vi "[Backup]BeamScanner.vi"() -> ()   [LabVIEW 2016]
uses:
  C:/Program Files/Ocean Optics/OmniDriver/OOI_HOME/NETOmniDriver-NET40.dll
  Program Files/Ocean Optics/OmniDriver/OOI_HOME/NETOmniDriver-NET40.dll
  <vilib>/DAQmx/write.llb/DAQmx Write (Digital Bool 1Line 1Point).vi
  <vilib>/DAQmx/write.llb/DAQmx Write (Analog DBL 1Chan 1Samp).vi
  <vilib>/DAQmx/write.llb/DAQmx Write (Analog 1D DBL NChan 1Samp).vi
  <vilib>/DAQmx/write.llb/DAQmx Write (Analog 2D DBL NChan NSamp).vi
  <vilib>/Analysis/baseanly.llb/Mean (DBL).vi
  <vilib>/DAQmx/read.llb/DAQmx Read (Raw 1D I16).vi
  <vilib>/DAQmx/create/channels.llb/DAQmx Create Channel (DO-Digital Output).vi
  <vilib>/DAQmx/miscellaneous.llb/DAQmx Fill In Error Info.vi
  <vilib>/DAQmx/create/channels.llb/DAQmx Create Channel (AO-Voltage-Basic).vi
  resources/MotorPosition.vi
  <vilib>/DAQmx/create/channels.llb/DAQmx Create Channel (AI-Voltage-Basic).vi
  <vilib>/DAQmx/configure/timing.llb/DAQmx Timing (Sample Clock).vi
  <vilib>/DAQmx/configure/trigger.llb/DAQmx Start Trigger (Digital Edge).vi
  <vilib>/Analysis/NI_AALBase.lvlib
  <resource>/objmgr/daqmx.rc
panel:
  in  "OCM Setup":bool
  in  "Home X":dbl=-121.7
  in  "Home  Y":dbl=-91.8
  in  "sampling rate (ADC)":u32(ring)=1250000 items=["500000"=500000, "750000"=750000, "1000000"=1000000, "1250000"=1250000]
  in  "Intgration time [us]":u32=44444 min=7000 max=10000000 step=1
  in  "Wavelength max":dbl=761.0 min=200.0 max=1100.0 step=1.0
  in  "Wavelength min":dbl=374.0 min=200.0 max=1100.0 step=1.0 format="%#.4g"
  out "spectral image":u32[][][](array[numeric])
  out "read task":refnum<k21>
  out "write task":refnum<k21>
  in  "Detector":u16(ring) items=["PMT", "QEPro", "Basler OCM"]
  out "scanning waveforms":dbl[][](array[numeric])
  out "Retrace":dbl[][](array[numeric])
  in  "Move to z":bool
  out "z-Position":sgl format="%.2g"
  out "xy-Position [µm]":sgl[](array[numeric]) min=0 max=500
  in  "Thrown samples":i16=500
  in  "Throw away":bool
  out "Samples/Pixel":u32
  in  "PMT output range":dbl(ring)=10.0 items=["-0,1V – 0,1V"=0.1, "-0,2V – 0,2V"=0.2, "-0,5V – 0,5V"=0.5, "-1V – 1V"=1.0, "-2V – 2V"=2.0, "-5V – 5V"=5.0, "-10V – 10V"=10.0]
  out "Time of last scan memory":string
  out "Info File contents memory":string
  out "Info File contents":string
  out "Time per line [s]":dbl format="%#.1g"
  out "Time of last scan":string
  out "scaling factor (length/voltage)":dbl
  in  "Additional info":string
  in  "Save":bool
  in  "Quit":bool
  in  "PMT sensitivity":dbl min=-1989.12 max=1989.12 format="%#.2f"
  in  "requested z-Position":dbl min=0.0 max=10.0
  in  "# steps":u16=20 step=1 format="%#.0f"
  out "Duration (m.s)":string
  in  "Scanrate (pixels/s)":u32(ring)=10000 items=["250 kHz"=250000, "125 kHz"=125000, "50 kHz (!)"=50000, "25 kHz (!)"=25000, "10 kHz (?)"=10000, "5 kHz (?)"=5000, "2 kHz"=2000, "1 kHz"=1000, "500 Hz"=500, "200 Hz"=200, "100 Hz"=100]
  out "Optimal":string
  out "Optimal pixel size [nm]":dbl format="%#.0f"
  in  "NA":dbl=1.0 min=0.0
  in  "Swap Memory":bool
  out "Memory":dbl[][](graph)
  out "System":bool
  in  "Use white point":bool
  in  "Magnification":dbl=20.0
  in  "Go home":bool
  in  "Go to white point":bool
  in  "z-Maximum val":dbl min=0.0 max=500.0 format="%#.2f"
  in  "z-Minimum val":dbl min=0.0 max=500.0 format="%#.2f"
  in  "z-Stacking":bool
  in  "Step size":dbl=1.0 min=0.0
  in  "z-Minimum":dbl(slide) min=0.0 max=500.0 step=1.0 scale=0.0..500.0
  in  "z-Maximum":dbl(slide)=0.30612244897959184 min=96.0 max=500.0 step=1.0 scale=0.0..500.0
  out "Path":path
  in  "File identifier":string="unnamed_file"
  in  "Save Image":bool
  in  "Scan":bool
  in  "y-Offset":dbl min=-480.0 max=480.0 format="%#.2f"
  in  "x-Offset":dbl min=-480.0 max=480.0 format="%#.2f"
  in  "Field of View":dbl(ring)=0.471281296023564 items=["4x4 µm"=0.02945508100147275, "8x8 µm"=0.0589101620029455, "16x16 µm"=0.117820324005891, "32x32 µm"=0.235640648011782, "64x64 µm"=0.471281296023564, "128x128 µm"=0.942562592047128, "256x256 µm"=1.885125184094256, "512x512 µm"=3.770250368188512, "1024x1024 µm"=7.540500736377024, "0x0"=0.0]
  out "Image":dbl[][](graph)
  in  "Number of pixels":i32(ring)=128 items=["8x8"=8, "16x16"=16, "32x32"=32, "64x64"=64, "128x128"=128, "256x256"=256, "512x512"=512, "1024x1024"=1024, "optimal"=640]
  # "make setup button"
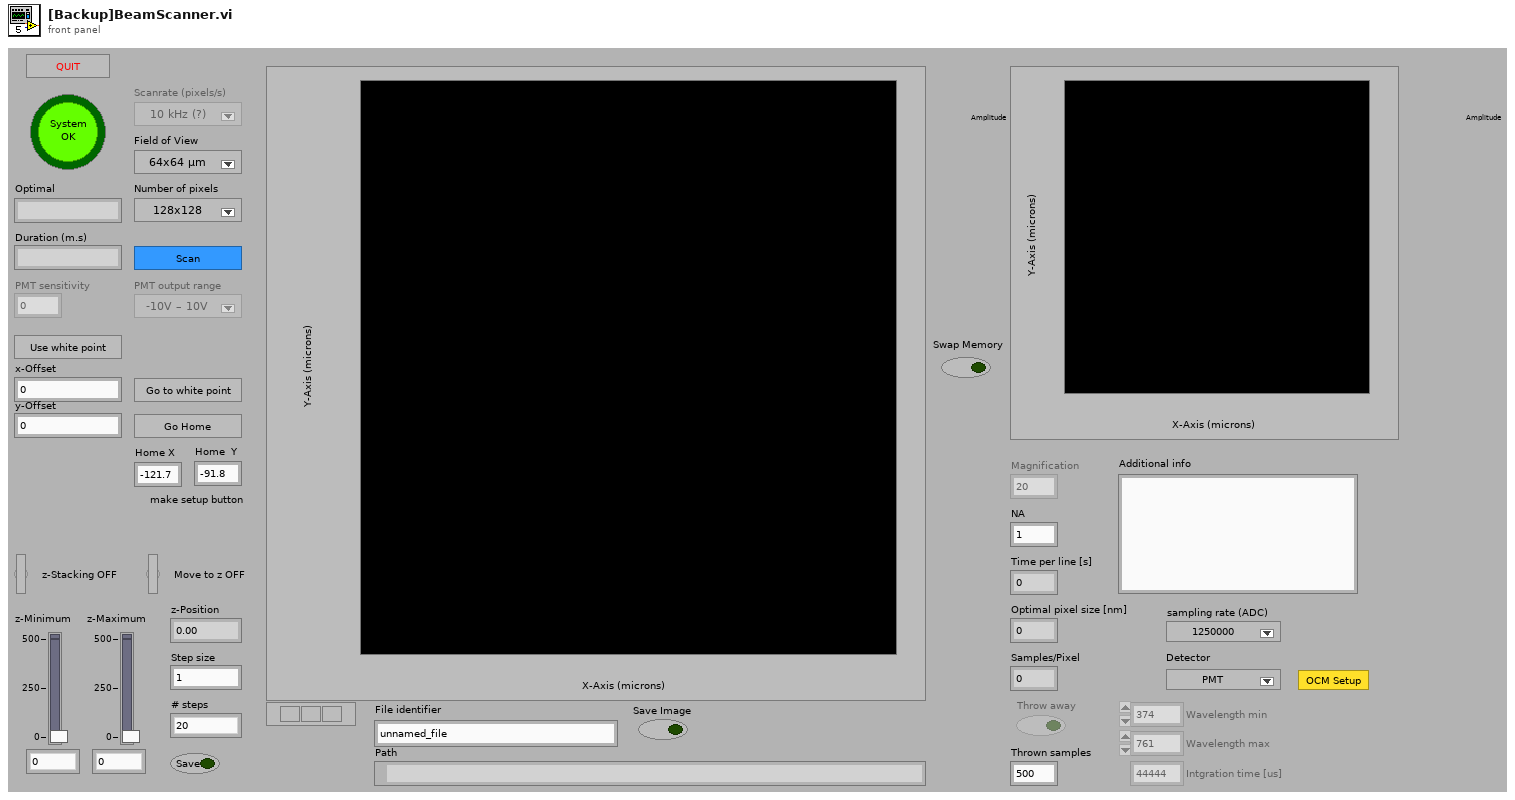
[diagram p1: front panel]
types:
  T1 = enum8{"Enabled", "Disabled", "Disabled and Grayed Out"}
  T2 = typedef "LVStringsAndValuesArrayTypeDef_DBL.ctl" = cluster{"String":string, "Value":dbl}[]
  T3 = typedef "LVStringsAndValuesArrayTypeDef_I32.ctl" = cluster{"String":string, "Value":i32}[]
  T4 = typedef "LVOffsetAndMultiplierTypeDef.ctl" = cluster{"Offset":dbl, "Multiplier":dbl}
  T5 = typedef "Maya2000 basic info.ctl" = cluster{"This instruments index":i32, "Name+SerialNumber":string, "Number Dark pixels":i32, "NumberOfPixels\nper spectrum":i32, "NumberOf Maya2000 instrm.":i32, "MaximumIntegrationTime\n[us]":i32, "MinimumIntegrationTime\n[us]":i32}
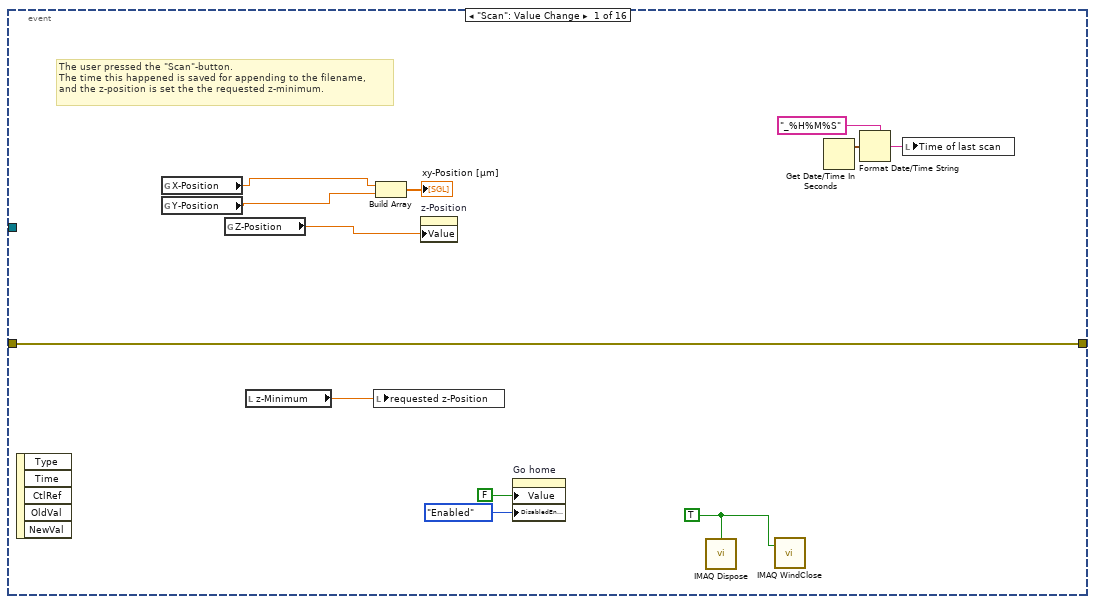
[diagram p2: hidden frame]
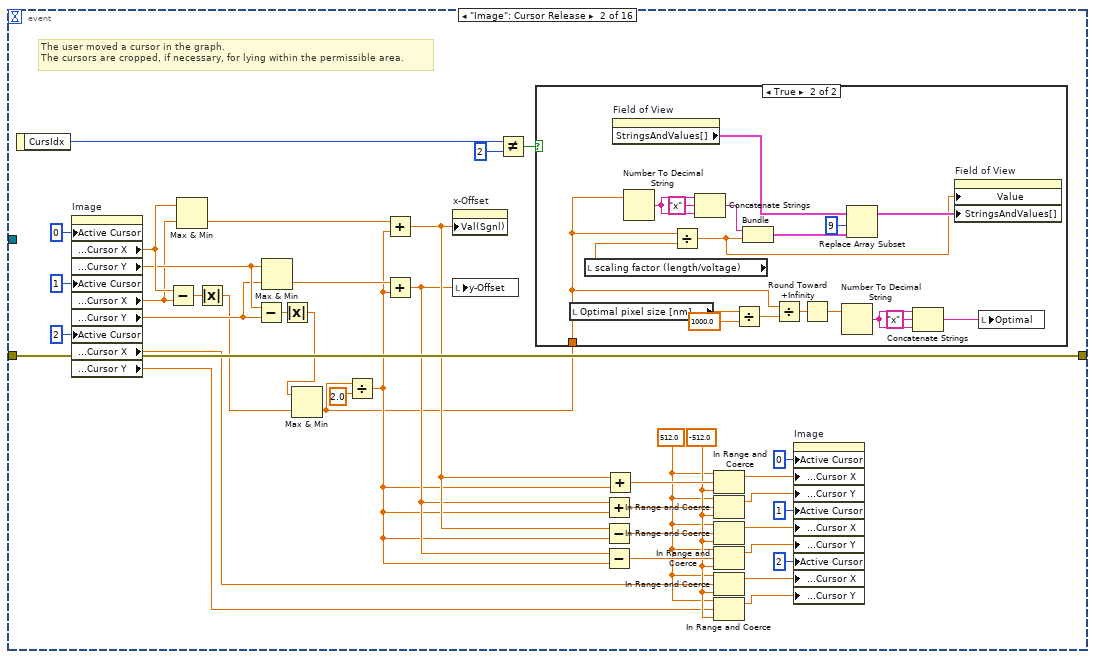
[diagram p3: hidden frame]
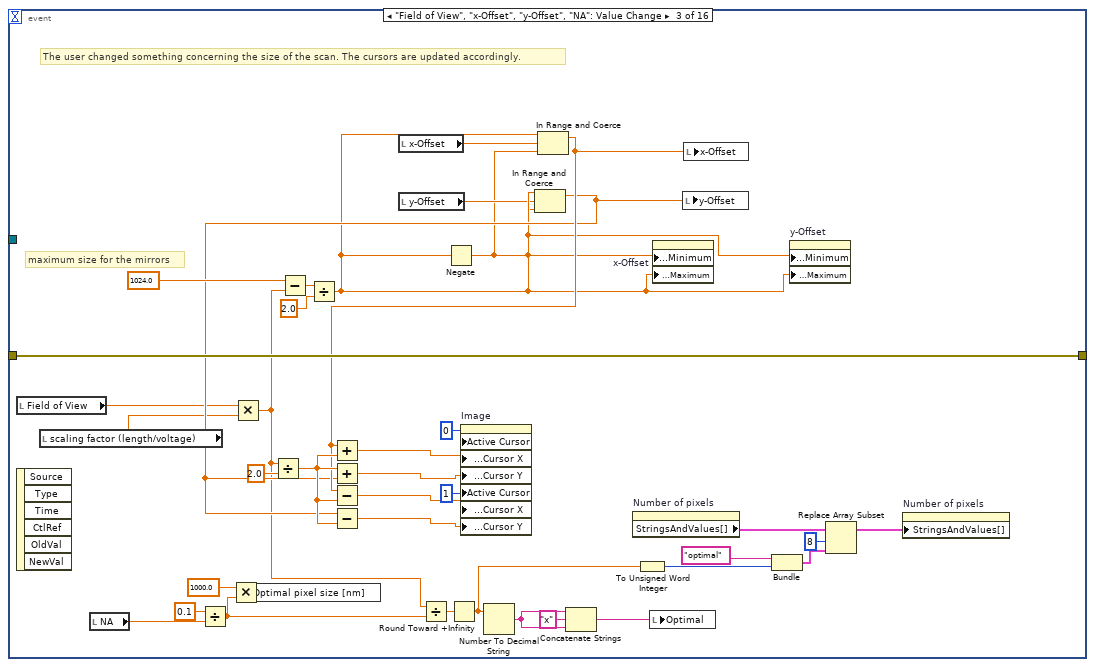
[diagram p5: hidden frame]
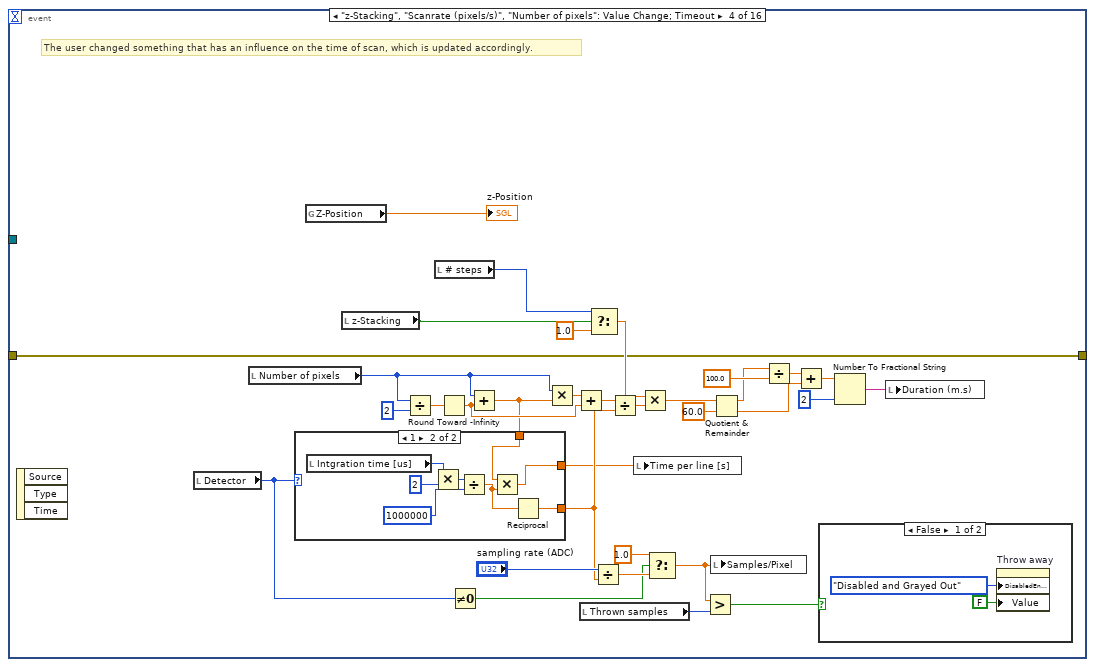
[diagram p6: hidden frame]
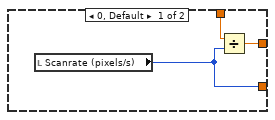
[diagram p7: hidden frame]
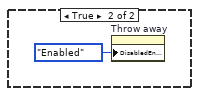
[diagram p8: hidden frame]
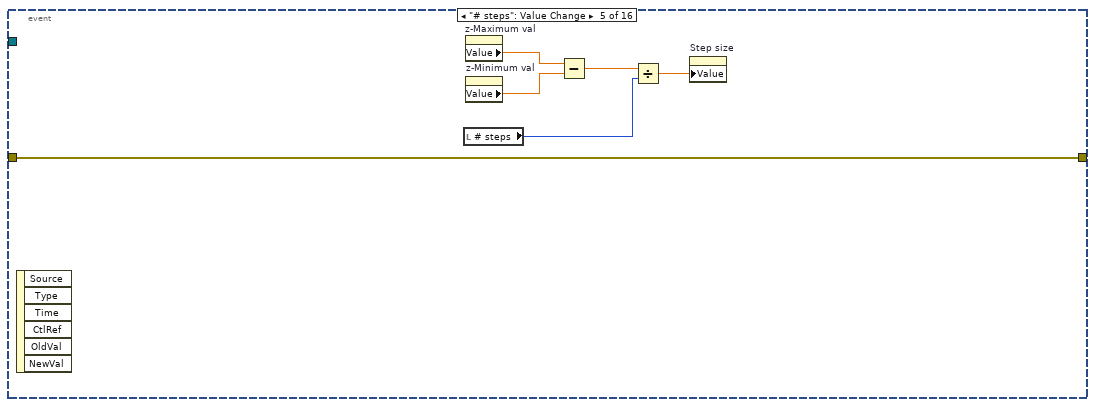
[diagram p9: hidden frame]
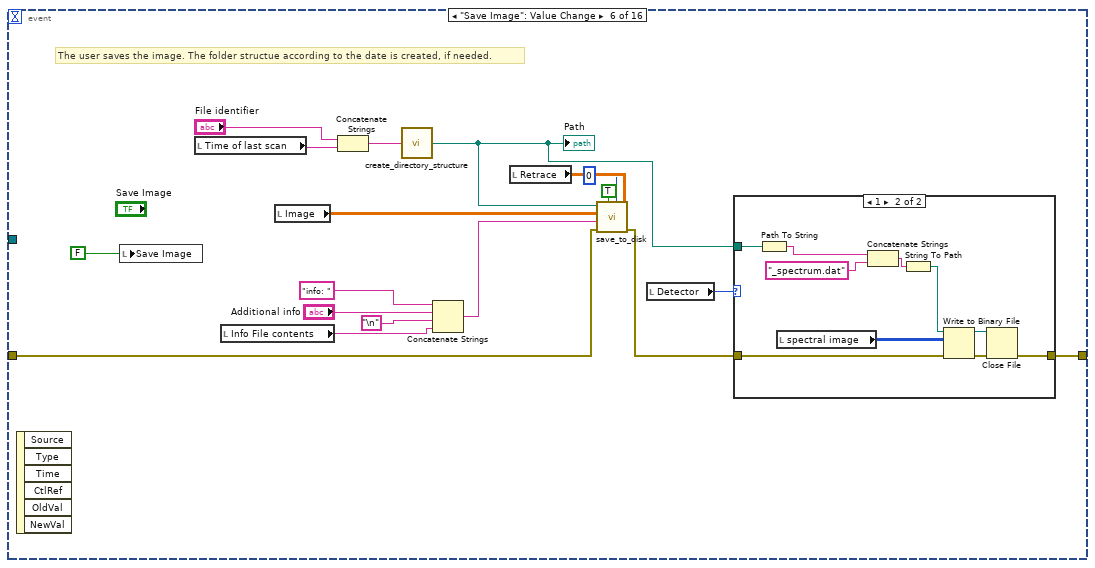
[diagram p10: hidden frame]
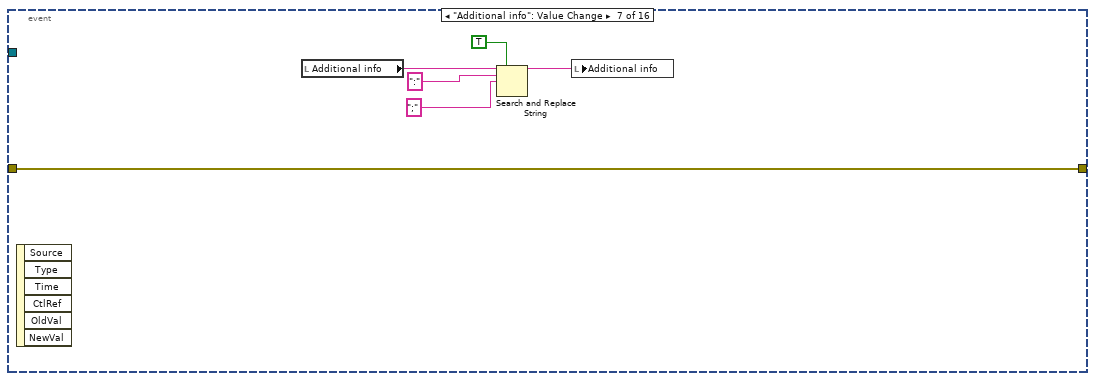
[diagram p12: hidden frame]
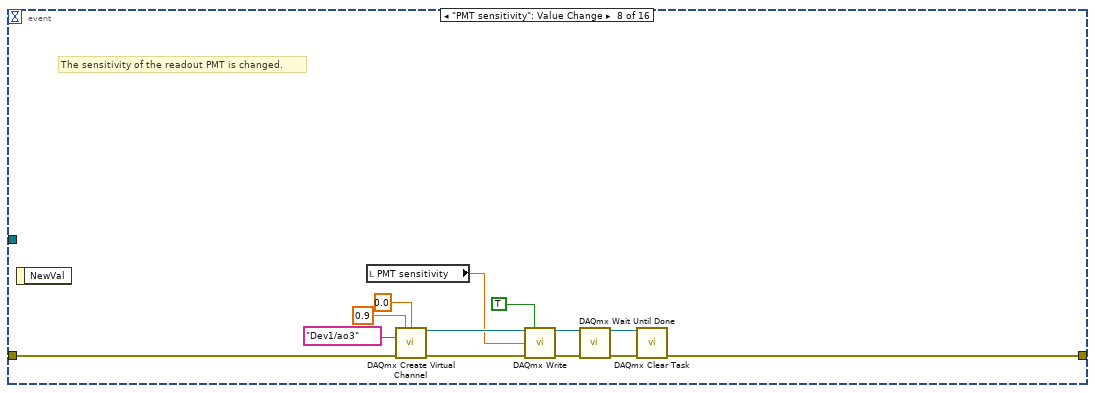
[diagram p13: hidden frame]
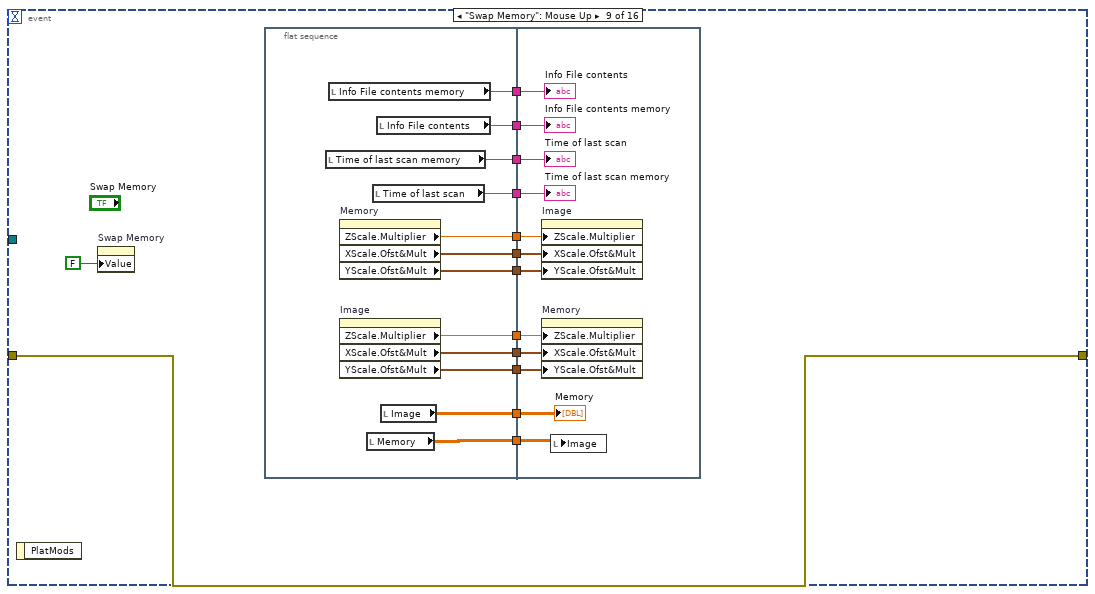
[diagram p14: hidden frame]
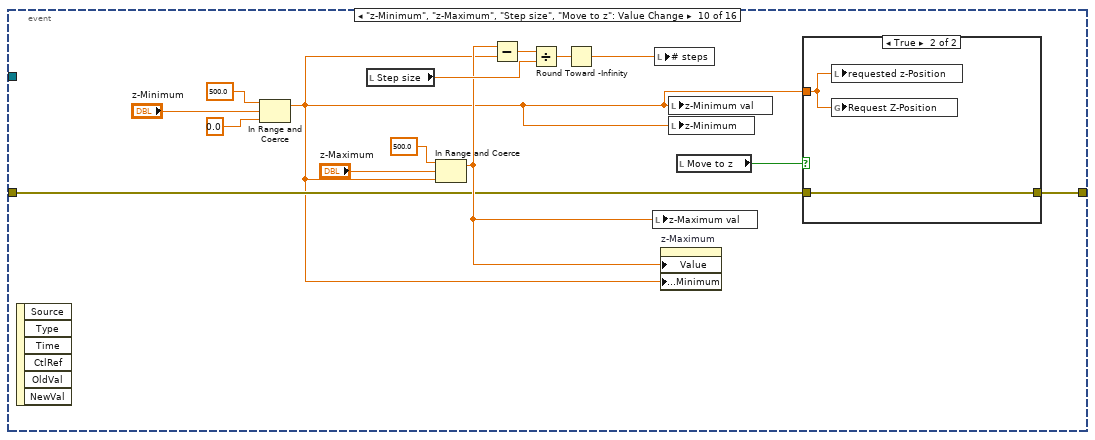
[diagram p15: hidden frame]
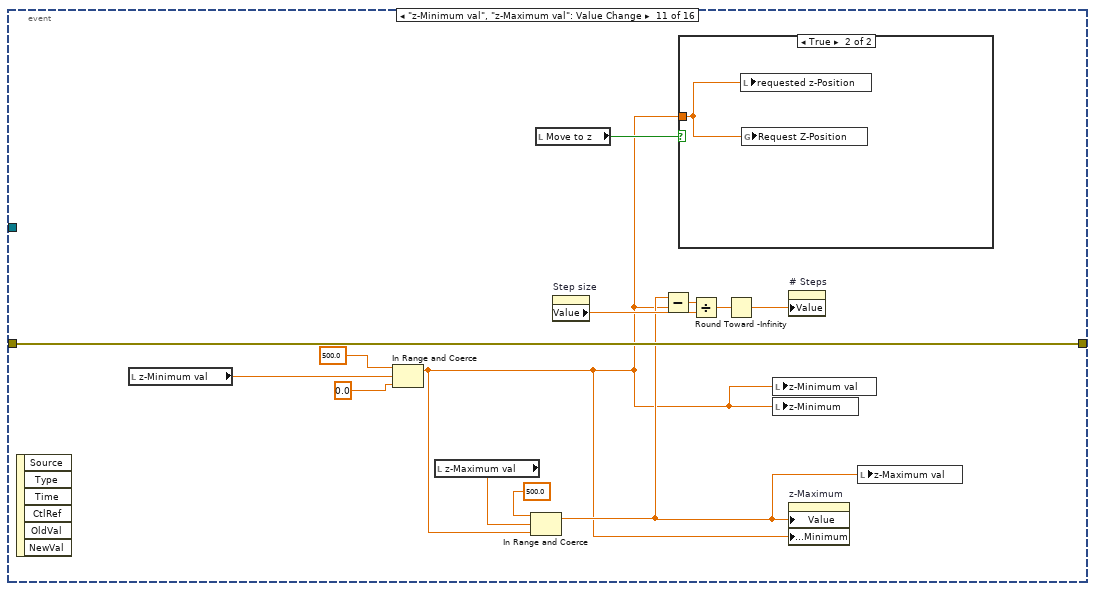
[diagram p17: hidden frame]
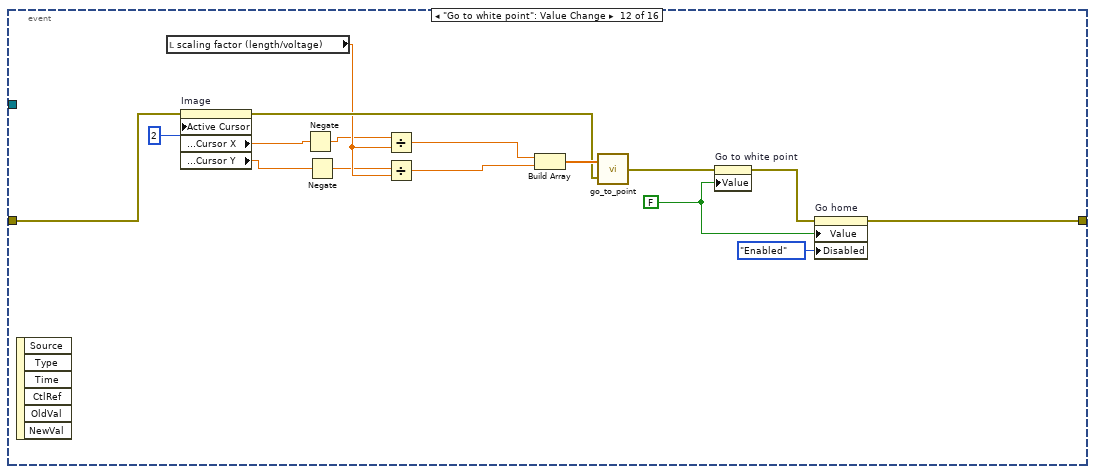
[diagram p19: hidden frame]
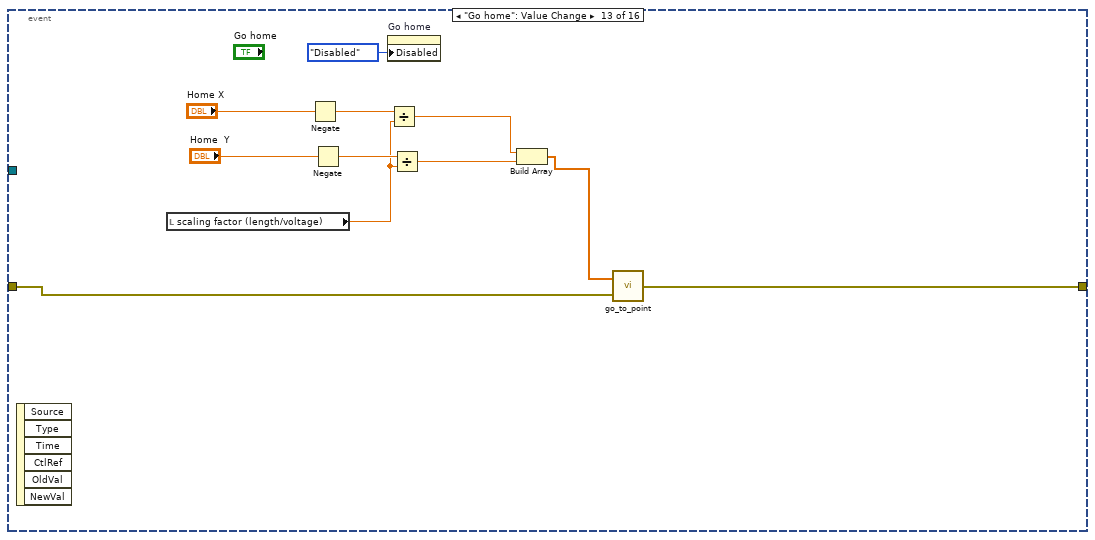
[diagram p20: hidden frame]
diagram:
  w2 = FALSE ("Visible")
  w24 = 0.0 ("y-Offset")
  w13 = FALSE ("System")
  # "These are local variable containers,\ninvisible to the user"
  # "Close the shutter"
  # "First, we initialise a few values, e.g.\nthe \"Save Image\" button is hidden,\nand the \"Scan\" button is set to false."
  n1 = call-poly <vilib>:"DAQmx Create Virtual Channel.vi"("lines"=tag "Dev1/port2/line0") -> ("task out"=w62:refnum<k21>, "error out"=w61:errorcluster)  [unwired: 13 in]
  n2 = property on="System" class="Bool (strict)"("Value"=TRUE ("System")) -> ()  [unwired: 2 in, 2 out]
  n3 = property on="Go to white point" class="Bool (strict)"("Value"=w13) -> ()  [unwired: 2 in, 2 out]
  n4 = property on="Quit" class="Bool (strict)"("Value"=w13) -> ()  [unwired: 2 in, 2 out]
  n5 = property on="Scan" class="Bool (strict)"("Value"=w13) -> ()  [unwired: 2 in, 2 out]
  n6 = property on="Go home" class="Bool (strict)"("Value"=w13, "DisabledEnum"=T1."Enabled" ("Disabled")) -> ()  [unwired: 2 in, 2 out]
  n7 = local write "x-Offset"(w24) -> ()
  n8 = local write "y-Offset"(w24) -> ()
  n9 = property on="OCM Setup" class="Bool"("Visible"=FALSE) -> ()  [unwired: 2 in, 2 out]
  n10 = call-poly <vilib>:"DAQmx Write.vi"("task/channels in"=w62, "data"=FALSE, "error in"=w61) -> ("task out"=w59:refnum<k21>, "error out"=w58:errorcluster)  [unwired: 10 in, 1 out]
  n11 = property on="Magnification" class="DigNum (strict)"("DisabledEnum"=T1."Disabled and Grayed Out" ("Disabled")) -> ()  [unwired: 2 in, 2 out]
  n12 = call <vilib>:"DAQmx Clear Task.vi"("task in"=w59, "error in"=w58) -> ("error out"=w46:errorcluster)  [unwired: 13 in]
  n13 = property on="write task" class="DAQmxName (strict)"("Visible"=w2) -> ()  [unwired: 2 in, 2 out]
  n14 = property on="read task" class="DAQmxName (strict)"("Visible"=w2) -> ()  [unwired: 2 in, 2 out]
  n15 = property on="scanning waveforms" class="Arr (strict)"("Visible"=w2) -> ()  [unwired: 2 in, 2 out]
  n16 = property on="Retrace" class="Arr (strict)"("Visible"=w2) -> ()  [unwired: 2 in, 2 out]
  n17 = property on="info file contents" class="Str"("Visible"=w2) -> ()  [unwired: 2 in, 2 out]
  n18 = property on="time of last scan" class="Str"("Visible"=w2) -> ()  [unwired: 2 in, 2 out]
  n19 = property on="info file contents memory" class="Str"("Visible"=w2) -> ()  [unwired: 2 in, 2 out]
  n20 = property on="time of last scan memory" class="Str"("Visible"=w2) -> ()  [unwired: 2 in, 2 out]
  n21 = property on="scaling factor (length/voltage)" class="DigNum (strict)"("Visible"=w2) -> ()  [unwired: 2 in, 2 out]
  n22 = property on="xy-Position [µm]" class="Arr (strict)"("Visible"=w2) -> ()  [unwired: 2 in, 2 out]
  n23 = property on="spectral image" class="Arr (strict)"("Visible"=w2) -> ()  [unwired: 2 in, 2 out]
  n24 = property on="requested z-Position" class="DigNum (strict)"("Visible"=w2) -> ()  [unwired: 2 in, 2 out]
  n25 = Divide(x=0.1, y="NA") -> (x/y=w35:dbl)
  n26 = call-poly <vilib>:"DAQmx Create Virtual Channel.vi"("maximum value"=0.9, "minimum value"=0.0, "physical channels"=tag "Dev1/ao3", "error in"=w46) -> ("task out"=w50:refnum<k21>, "error out"=w49:errorcluster)  [unwired: 10 in]
  n27 = Divide(x=2716.0, y="Magnification") -> (x/y=w20:dbl)
  "scaling factor (length/voltage)" <- w20
  n28 = Multiply(x=1000.0, y=w35) -> (x*y=→"Optimal pixel size [nm]":dbl)
  n29 = call-poly <vilib>:"DAQmx Write.vi"("task/channels in"=w50, "auto start"=TRUE, "data"="PMT sensitivity", "error in"=w49) -> ("task out"=w53:refnum<k21>, "error out"=w52:errorcluster)  [unwired: 9 in, 1 out]
  n30 = for {
    N: 8 -> [_]
    tunnel: [w77] -> w29 mode=indexing
    i -> [w84]
    n31 = Add(x=3, y=w84) -> (x+y=w81:i32)
    n32 = Scale By Power Of 2(n=w81, x=u16 1) -> (x*2^n=w78:u16)
    n33 = Format Into String(format string="%dx%d", w78, w78) -> (resulting string=w79:string)  [unwired: 2 in, 1 out]
    n34 = Bundle(w79, w78) -> (w77:cluster{string, u16})  [unwired: 1 in]
  }
  n35 = call <vilib>:"DAQmx Wait Until Done.vi"("task/channels in"=w53, "error in"=w52) -> ("task out"=w48:refnum<k21>, "error out"=w47:errorcluster)  [unwired: 12 in]
  n36 = Multiply(x=w20, y="Field of View") -> (x*y=w39:dbl)
  n37 = call <vilib>:"DAQmx Clear Task.vi"("task in"=w48, "error in"=w47) -> ("error out"=w45:errorcluster)  [unwired: 13 in]
  n38 = Divide(x=w39, y=w35) -> (x/y=w38:dbl)
  n39 = Build Array(tag "Dev1/ao0" ("physical channels"), tag "Dev1/ao1" ("physical channels")) -> (w74:tag[])
  n40 = Round Toward +Infinity(x=w38) -> (ceil(x): smallest int >= x=w31:dbl)
  n41 = call <vilib>:"DAQmx Flatten Channel String.vi"("names in"=w74, "error in"=w45) -> ("names out"=w73:string, "error out"=w72:errorcluster)  [unwired: 12 in]
  n42 = Number To Decimal String(number=w31) -> (decimal integer string=w36:string)  [unwired: 1 in]
  n43 = To Unsigned Word Integer(number=w31) -> (unsigned 16bit integer=w30:u16)
  n44 = call-poly <vilib>:"DAQmx Create Virtual Channel.vi"("physical channels"=w73, "error in"=w72) -> ("task out"=w70:refnum<k21>, "error out"=w69:errorcluster)  [unwired: 12 in]
  n45 = for {
    N: 9 -> [_]
    tunnel: w20 -> [w87]
    tunnel: [w86] -> w18 mode=indexing
    i -> [w91]
    n46 = Add(x=2, y=w91) -> (x+y=w93:i32)
    n47 = Scale By Power Of 2(n=w93, x=u16 1) -> (x*2^n=w88:u16)
    n48 = Divide(x=w88, y=w87) -> (x/y=w85:dbl)
    n49 = Format Into String(format string="%dx%d \\B5m", w88, w88) -> (resulting string=w89:string)  [unwired: 2 in, 1 out]
    n50 = Bundle(w89, w85) -> (w86:cluster{string, dbl})  [unwired: 1 in]
  }
  n51 = Concatenate Strings(w36, "x" ("string"), w36) -> (→"Optimal":string)
  n52 = call-poly <vilib>:"DAQmx Write.vi"("task/channels in"=w70, "data"=dbl[] [0.0, 0.0], "error in"=w69) -> ("task out"=w67:refnum<k21>, "error out"=w65:errorcluster)  [unwired: 10 in, 1 out]
  n53 = Bundle("string"="optimal", w30) -> (w28:cluster{"string":string, u16})  [unwired: 1 in]
  n54 = call <vilib>:"DAQmx Wait Until Done.vi"("task/channels in"=w67, "error in"=w65) -> ("task out"=w66:refnum<k21>, "error out"=w64:errorcluster)  [unwired: 12 in]
  n55 = Build Array (concatenate)(w29, w28) -> (w27:cluster{"string":string, u16}[])
  n56 = call <vilib>:"DAQmx Clear Task.vi"("task in"=w66, "error in"=w64) -> ("error out"=w5:errorcluster)  [unwired: 13 in]
  n57 = property on="Number of pixels" class="Ring (strict)"("StringsAndValues[]"=w27) -> ()  [unwired: 2 in, 2 out]
  n58 = Open VI Reference(vi path=path "kinesis/kinesis.vi", error in (no error)=w5) -> (vi reference=w11:refnum<vi>, error out=w10:errorcluster)  [unwired: 4 in]
  n59 = invoke class="VI" method="Run VI"(reference=w11, error in=w10, "Wait until done"=FALSE ("Wait Until Done")) -> (reference out=w8:refnum<vi>, error out=w7:errorcluster)  [unwired: 2 in, 3 out]
  n60 = Bundle("format string"="0x0", 0.0) -> (w17:cluster{"format string":string, dbl})  [unwired: 1 in]
  n61 = Build Array (concatenate)(w18, w17) -> (w14:cluster{"format string":string, dbl}[])
  n62 = property on="Field of View" class="Ring (strict)"("Strings And Values []"=w14) -> ()  [unwired: 2 in, 2 out]
  n63 = invoke class="VI" method="FP.Open"(reference=w8, error in=w7, "Activate"=TRUE ("Activate?")) -> (reference out=w3:refnum<vi>, error out=w4:errorcluster)  [unwired: 2 in, 3 out]
  n64 = while {
    shift-right: [w97] -> w19
    shift-left: w4 -> [w103]
    tunnel: w3 -> [w95]
    stop <- w98 stop-if-true
    n65 = flat-sequence {
      tunnel: w103 -> [w107]
      tunnel: [w106] -> w104
      tunnel: w95 -> [w105]
      tunnel: w104 -> [w507]
      tunnel: [w507] -> w102
      tunnel: w102 -> [w550]
      tunnel: [w549] -> w101
      tunnel: w101 -> [w569]
      tunnel: [w568] -> w96
      tunnel: [w633] -> w100
      tunnel: [w632] -> w99
      tunnel: w96 -> [w631]
      tunnel: w100 -> [w1019]
      tunnel: w99 -> [w1016]
      tunnel: [w1017] -> w97
      tunnel: [w1020] -> w98
      frame #0 {
        n66 = while {
          shift-right: [w113] -> w106
          shift-left: w107 -> [w115]
          tunnel: w105 -> [w108]
          stop <- w112 stop-if-true
          # "The individual routines are called via events. The program waits, until an event occurs."
          n67 = event shown="[14] \"Detector\": Value Change" {
            selector: _ -> [_ _ _ _ _ _ _ _ _ _ _ _ _ _ _ _]
            dyn-events: _ -> [_ _ _ _ _ _ _ _ _ _ _ _ _ _ _ _]
            timeout: 100 -> [_ _ _ _ _ _ _ _ _ _ _ _ _ _ _ _]
            tunnel: w115 -> [w121 w149 w208 w231 w269 w280 w304 w312 w327 w363 w384 w401 w418 w433 w446 w460]
            tunnel: [w121 w149 w208 w231 w269 w276 w304 w311 w327 w362 w384 w400 w417 w433 w446 w461] -> w113
            tunnel: w108 -> [_ _ _ _ _ _ _ _ _ _ _ _ _ _ _ w458]
            event "Scan": Value Change {
              w120 = TRUE ("All Images? (No)")
              # "The user pressed the \"Scan\"-button.\nThe time this happened is saved for appending to the filename,\nand the z-position is set the the requested z-minimum."
              n68 = event-data() -> ()  [unwired: 1 in, 5 out]
              n69 = global read "MotorPosition.vi" "X-Position"() -> (w117:dbl)
              n70 = global read "MotorPosition.vi" "Y-Position"() -> (w116:dbl)
              n71 = global read "MotorPosition.vi" "Z-Position"() -> (w119:dbl)
              n72 = local read "z-Minimum"() -> (w122:dbl)
              n73 = local write "requested z-Position"(w122) -> ()
              n74 = Build Array(w117, w116) -> (→"xy-Position [µm]":dbl[])
              n75 = property on="z-Position" class="DigNum (strict)"("Value"=w119) -> ()  [unwired: 2 in, 2 out]
              n76 = property on="Go home" class="Bool (strict)"("Value"=FALSE ("Go home"), "DisabledEnum"=T1."Enabled" ("Disabled")) -> ()  [unwired: 2 in, 2 out]
              n77 = call "IMAQ Dispose"("All Images? (No)"=w120) -> ()  [unwired: 5 in, 1 out]
              n78 = call "IMAQ WindClose"("Close All Windows (False)"=w120) -> ()  [unwired: 5 in, 1 out]
              n79 = Get Date/Time In Seconds() -> (seconds since 1Jan1904=w126:timestamp)
              n80 = Format Date/Time String(time format string (%c)="_%H%M%S", seconds (now)=w126) -> (date/time string=w123:string)  [unwired: 1 in]
              n81 = local write "Time of last scan"(w123) -> ()
            }
            event "Image": Cursor Release {
              w150 = 512.0 ("upper limit")
              w151 = -512.0 ("upper limit")
              # "The user moved a cursor in the graph.\nThe cursors are cropped, if necessary, for lying within the permissible area."
              n82 = event-data() -> ("CursIdx"=w129:i32)  [unwired: 1 in]
              n83 = property on="Image" class="IntGraph (strict)"("Active Cursor"=u32 0, "Active Cursor"=u32 1, "Active Cursor"=u32 2) -> ("Cursor.Cursor Position:Cursor X"=w148:dbl, "Cursor.Cursor Position:Cursor Y"=w147:dbl, "Cursor.Cursor Position:Cursor X"=w146:dbl, "Cursor.Cursor Position:Cursor Y"=w145:dbl, "Cursor.Cursor Position:Cursor X"=w144:dbl, "Cursor.Cursor Position:Cursor Y"=w143:dbl)  [unwired: 2 in, 2 out]
              n84 = Subtract(x=w148, y=w146) -> (x-y=w164:dbl)
              n85 = Max & Min(x=w148, y=w146) -> (min(x,y)=w161:dbl)  [unwired: 1 out]
              n86 = Absolute Value(x=w164) -> (abs(x)=w141:dbl)
              n87 = Subtract(x=w147, y=w145) -> (x-y=w163:dbl)
              n88 = Max & Min(x=w147, y=w145) -> (min(x,y)=w160:dbl)  [unwired: 1 out]
              n89 = Absolute Value(x=w163) -> (abs(x)=w142:dbl)
              n90 = Max & Min(x=w142, y=w141) -> (min(x,y)=w131:dbl)  [unwired: 1 out]
              n91 = Divide(x=w131, y=2.0) -> (x/y=w132:dbl)
              n92 = Add(x=w161, y=w132) -> (x+y=w140:dbl)
              n93 = Add(x=w160, y=w132) -> (x+y=w133:dbl)
              n94 = property on="x-Offset" class="DigNum (strict)"("Val(Sgnl)"=w140) -> ()  [unwired: 2 in, 2 out]
              n95 = local write "y-Offset"(w133) -> ()
              n96 = Not Equal?(x=w129, y=2) -> (x != y?=w130:bool)
              n97 = case shown="True" w130 {
                tunnel: w131 -> [_ w173]
                frame False {
                  # "The user moved the white cursor, so no updating is required"
                }
                frame True {
                  n98 = local read "Optimal pixel size [nm]"() -> (w177:dbl)
                  n99 = local read "scaling factor (length/voltage)"() -> (w176:dbl)
                  n100 = property on="Field of View" class="Ring (strict)"() -> ("StringsAndValues[]"=w172:T2)  [unwired: 2 in, 2 out]
                  n101 = Number To Decimal String(number=w173) -> (decimal integer string=w174:string)  [unwired: 1 in]
                  n102 = Divide(x=w173, y=w176) -> (x/y=w167:dbl)
                  n103 = Concatenate Strings(w174, "x" ("string"), w174) -> (w169:string)
                  n104 = Divide(x=w177, y=1000.0 ("x")) -> (x/y=w180:dbl)
                  n105 = Bundle(w169, w167) -> (w171:cluster{string, dbl})  [unwired: 1 in]
                  n106 = Divide(x=w173, y=w180) -> (x/y=w184:dbl)
                  n107 = Round Toward +Infinity(x=w184) -> (ceil(x): smallest int >= x=w183:dbl)
                  n108 = Number To Decimal String(number=w183) -> (decimal integer string=w181:string)  [unwired: 1 in]
                  n109 = Replace Array Subset(array=w172, new element=w171, index=9) -> (w168:T2)
                  n110 = Concatenate Strings(w181, "x" ("string"), w181) -> (w179:string)
                  n111 = property on="Field of View" class="Ring (strict)"("Value"=w167, "StringsAndValues[]"=w168) -> ()  [unwired: 2 in, 2 out]
                  n112 = local write "Optimal"(w179) -> ()
                }
              }
              n113 = Add(x=w133, y=w132) -> (x+y=w156:dbl)
              n114 = Subtract(x=w140, y=w132) -> (x-y=w155:dbl)
              n115 = Subtract(x=w133, y=w132) -> (x-y=w154:dbl)
              n116 = Add(x=w140, y=w132) -> (x+y=w157:dbl)
              n117 = In Range and Coerce(upper limit=w150, x=w157, lower limit=w151) -> (coerced(x)=w139:dbl)  [unwired: 1 out]
              n118 = In Range and Coerce(upper limit=w150, x=w156, lower limit=w151) -> (coerced(x)=w138:dbl)  [unwired: 1 out]
              n119 = In Range and Coerce(upper limit=w150, x=w155, lower limit=w151) -> (coerced(x)=w137:dbl)  [unwired: 1 out]
              n120 = In Range and Coerce(upper limit=w150, x=w154, lower limit=w151) -> (coerced(x)=w136:dbl)  [unwired: 1 out]
              n121 = In Range and Coerce(upper limit=w150, x=w144, lower limit=w151) -> (coerced(x)=w135:dbl)  [unwired: 1 out]
              n122 = In Range and Coerce(upper limit=w150, x=w143, lower limit=w151) -> (coerced(x)=w134:dbl)  [unwired: 1 out]
              n123 = property on="Image" class="IntGraph (strict)"("Active Cursor"=u32 0, "Cursor.Cursor Position:Cursor X"=w139, "Cursor.Cursor Position:Cursor Y"=w138, "Active Cursor"=u32 1, "Cursor.Cursor Position:Cursor X"=w137, "Cursor.Cursor Position:Cursor Y"=w136, "Active Cursor"=u32 2, "Cursor.Cursor Position:Cursor X"=w135, "Cursor.Cursor Position:Cursor Y"=w134) -> ()  [unwired: 2 in, 2 out]
            }
            event "Field of View", "x-Offset", "y-Offset", "NA": Value Change {
              # "The user changed something concerning the size of the scan. The cursors are updated accordingly."
              # "maximum size for the mirrors"
              n124 = local read "Field of View"() -> (w186:dbl)
              n125 = event-data() -> ()  [unwired: 1 in, 6 out]
              n126 = local read "scaling factor (length/voltage)"() -> (w190:dbl)
              n127 = local read "NA"() -> (w207:dbl)
              n128 = Divide(x=0.1, y=w207) -> (x/y=w210:dbl)
              n129 = Multiply(x=1000.0, y=w210) -> (x*y=w206:dbl)
              n130 = Multiply(x=w186, y=w190) -> (x*y=w185:dbl)
              n131 = local write "Optimal pixel size [nm]"(w206) -> ()
              n132 = Divide(x=w185, y=2.0) -> (x/y=w221:dbl)
              n133 = Subtract(x=1024.0, y=w185) -> (x-y=w216:dbl)
              n134 = Divide(x=w216, y=2.0) -> (x/y=w191:dbl)
              n135 = local read "x-Offset"() -> (w189:dbl)
              n136 = local read "y-Offset"() -> (w188:dbl)
              n137 = Divide(x=w185, y=w210) -> (x/y=w213:dbl)
              n138 = Negate(x=w191) -> (-x=w187:dbl)
              n139 = Round Toward +Infinity(x=w213) -> (ceil(x): smallest int >= x=w204:dbl)
              n140 = Number To Decimal String(number=w204) -> (decimal integer string=w211:string)  [unwired: 1 in]
              n141 = In Range and Coerce(upper limit=w191, x=w188, lower limit=w187) -> (coerced(x)=w196:dbl)  [unwired: 1 out]
              n142 = Add(x=w221, y=w196) -> (x+y=w194:dbl)
              n143 = Subtract(x=w196, y=w221) -> (x-y=w192:dbl)
              n144 = In Range and Coerce(upper limit=w191, x=w189, lower limit=w187) -> (coerced(x)=w197:dbl)  [unwired: 1 out]
              n145 = Add(x=w197, y=w221) -> (x+y=w195:dbl)
              n146 = Subtract(x=w197, y=w221) -> (x-y=w193:dbl)
              n147 = property on="Image" class="IntGraph (strict)"("Active Cursor"=u32 0, "Cursor.Cursor Position:Cursor X"=w195, "Cursor.Cursor Position:Cursor Y"=w194, "Active Cursor"=u32 1, "Cursor.Cursor Position:Cursor X"=w193, "Cursor.Cursor Position:Cursor Y"=w192) -> ()  [unwired: 2 in, 2 out]
              n148 = Concatenate Strings(w211, "x" ("string"), w211) -> (w203:string)
              n149 = property on="Number of pixels" class="Ring (strict)"() -> ("StringsAndValues[]"=w200:T3)  [unwired: 2 in, 2 out]
              n150 = To Unsigned Word Integer(number=w204) -> (unsigned 16bit integer=w205:u16)
              n151 = local write "Optimal"(w203) -> ()
              n152 = property on="x-Offset" class="DigNum (strict)"("Data Range:Minimum"=w187, "Data Range:Maximum"=w191) -> ()  [unwired: 2 in, 2 out]
              n153 = local write "y-Offset"(w196) -> ()
              n154 = local write "x-Offset"(w197) -> ()
              n155 = Bundle("string"="optimal", w205) -> (w202:cluster{"string":string, u16})  [unwired: 1 in]
              n156 = property on="y-Offset" class="DigNum (strict)"("Data Range:Minimum"=w187, "Data Range:Maximum"=w191) -> ()  [unwired: 2 in, 2 out]
              n157 = Replace Array Subset(array=w200, new element=w202, index=8) -> (w201:T3)
              n158 = property on="Number of pixels" class="Ring (strict)"("StringsAndValues[]"=w201) -> ()  [unwired: 2 in, 2 out]
            }
            event "z-Stacking", "Scanrate (pixels/s)", "Number of pixels": Value Change; Timeout {
              # "The user changed something that has an influence on the time of scan, which is updated accordingly."
              n159 = event-data() -> ()  [unwired: 1 in, 3 out]
              n160 = local read "Detector"() -> (w225:u16)
              n161 = local read "Number of pixels"() -> (w230:i32)
              n162 = global read "MotorPosition.vi" "Z-Position"() -> (→"z-Position":dbl)
              n163 = local read "z-Stacking"() -> (w236:bool)
              n164 = Divide(x=w230, y=2) -> (x/y=w254:dbl)
              n165 = local read "# steps"() -> (w239:u16)
              n166 = Round Toward -Infinity(1:w254) -> (0:w252:dbl)
              n167 = Not Equal To 0?(x=w225) -> (x != 0?=w224:bool)
              n168 = Add(x=w230, y=w252) -> (x+y=w229:dbl)
              n169 = case shown="1" w225 {
                tunnel: [w257 w263] -> w234
                tunnel: w229 -> [w256 w264]
                tunnel: [w255 w262] -> w223
                frame 0, Default {
                  n170 = local read "Scanrate (pixels/s)"() -> (w257:u32)
                  n171 = Divide(x=w256, y=w257) -> (x/y=w255:dbl)
                }
                frame 1 {
                  n172 = local read "Intgration time [us]"() -> (w259:u32)
                  n173 = Multiply(x=w259, y=u32 2) -> (x*y=w260:u32)
                  n174 = Divide(x=w260, y=u32 1000000) -> (x/y=w261:dbl)
                  n175 = Multiply(x=w264, y=w261) -> (x*y=w262:dbl)
                  n176 = Reciprocal(x=w261) -> (1/x=w263:dbl)
                }
              }
              n177 = Multiply(x=w230, y=w229) -> (x*y=w253:dbl)
              n178 = Add(x=w253, y=w252) -> (x+y=w251:dbl)
              n179 = local read "Thrown samples"() -> (w232:i16)
              n180 = Select(t=w239, s=w236, f=1.0) -> (s? t:f=w248:dbl)
              n181 = Divide(x="sampling rate (ADC)", y=w234) -> (x/y=w228:dbl)
              n182 = Divide(x=w251, y=w234) -> (x/y=w249:dbl)
              n183 = local write "Time per line [s]"(w223) -> ()
              n184 = Multiply(x=w248, y=w249) -> (x*y=w242:dbl)
              n185 = Select(t=1.0, s=w224, f=w228) -> (s? t:f=w227:dbl)
              n186 = Greater?(x=w227, y=w232) -> (0:w233:bool)
              n187 = local write "Samples/Pixel"(w227) -> ()
              n188 = Quotient & Remainder(x=w242, y=60.0) -> (x-y*floor(x/y)=w240:dbl, floor(x/y)=w246:dbl)
              n189 = Divide(x=w240, y=100.0) -> (x/y=w241:dbl)
              n190 = Add(x=w241, y=w246) -> (x+y=w244:dbl)
              n191 = case shown="False" w233 {
                frame False {
                  n192 = property on="Throw away" class="Bool (strict)"("DisabledEnum"=T1."Disabled and Grayed Out" ("Disabled"), "Value"=FALSE ("Throw away")) -> ()  [unwired: 2 in, 2 out]
                }
                frame True {
                  n193 = property on="Throw away" class="Bool (strict)"("DisabledEnum"=T1."Enabled" ("Disabled")) -> ()  [unwired: 2 in, 2 out]
                }
              }
              n194 = Number To Fractional String(number=w244, precision (6)=i16 2) -> (F-format string=w238:string)  [unwired: 2 in]
              n195 = local write "Duration (m.s)"(w238) -> ()
            }
            event "# steps": Value Change {
              n196 = event-data() -> ()  [unwired: 1 in, 6 out]
              n197 = local read "# steps"() -> (w270:u16)
              n198 = property on="z-Maximum val" class="DigNum (strict)"() -> ("Value"=w274:dbl)  [unwired: 2 in, 2 out]
              n199 = property on="z-Minimum val" class="DigNum (strict)"() -> ("Value"=w273:dbl)  [unwired: 2 in, 2 out]
              n200 = Subtract(x=w274, y=w273) -> (x-y=w272:dbl)
              n201 = Divide(x=w272, y=w270) -> (x/y=w271:dbl)
              n202 = property on="Step size" class="DigNum (strict)"("Value"=w271) -> ()  [unwired: 2 in, 2 out]
            }
            event "Save Image": Value Change {
              # "The user saves the image. The folder structue according to the date is created, if needed."
              n203 = event-data() -> ()  [unwired: 1 in, 6 out]
              n204 = local write "Save Image"(FALSE ("Bild speichern ...")) -> ()
              n205 = local read "Time of last scan"() -> (w291:string)
              n206 = local read "Info File contents"() -> (w284:string)
              n207 = local read "Image"() -> (w289:dbl[][])
              n208 = Concatenate Strings("File identifier", w291) -> (w283:string)
              n209 = call "create_directory_structure.vi"("File identifier"=w283) -> ("File path"=w277:path)
              "Path" <- w277
              n210 = Concatenate Strings("info: " ("format string"), "Additional info", "\n", w284) -> (w288:string)
              n211 = local read "Retrace"() -> (w281:dbl[][])
              n212 = call "save_to_disk.vi"("Retrace"=w281, "slice"=0, "write info file?"=TRUE, "error in"=w280, "Scan info"=w288, "Image"=w289, "File path"=w277) -> ("error out"=w278:errorcluster)  [unwired: 2 in]
              n213 = local read "Detector"() -> (w275:u16)
              n214 = case shown="1" w275 {
                tunnel: w278 -> [w293 w302]
                tunnel: w277 -> [_ w301]
                tunnel: [w293 w294] -> w276
                frame 0, Default {
                }
                frame 1 {
                  n215 = Path To String(path=w301) -> (string=w298:string)
                  n216 = local read "spectral image"() -> (w303:u32[][][])
                  n217 = Concatenate Strings(w298, "_spectrum.dat" ("string")) -> (w300:string)
                  n218 = String To Path(string=w300) -> (path=w297:path)
                  n219 = Write to Binary File(file (use dialog)=w297, data=w303, error in=w302) -> (refnum out=w295:refnum<file>, error out=w296:errorcluster)  [unwired: 3 in, 1 out]
                  n220 = Close File(refnum=w295, error in=w296) -> (error out=w294:errorcluster)  [unwired: 1 out]
                }
              }
            }
            event "Additional info": Value Change {
              n221 = event-data() -> ()  [unwired: 1 in, 6 out]
              n222 = local read "Additional info"() -> (w305:string)
              n223 = Search and Replace String(replace all?=TRUE ("replace all? (F)"), input string=w305, search string=":", replace string=";") -> (result string=w306:string)  [unwired: 4 in, 3 out]
              n224 = local write "Additional info"(w306) -> ()
            }
            event "PMT sensitivity": Value Change {
              # "The sensitivity of the readout PMT is changed."
              n225 = event-data() -> ()  [unwired: 1 in, 1 out]
              n226 = local read "PMT sensitivity"() -> (w310:dbl)
              n227 = call-poly <vilib>:"DAQmx Create Virtual Channel.vi"("maximum value"=0.9, "minimum value"=0.0, "physical channels"=tag "Dev1/ao3", "error in"=w312) -> ("task out"=w316:refnum<k21>, "error out"=w315:errorcluster)  [unwired: 10 in]
              n228 = call-poly <vilib>:"DAQmx Write.vi"("task/channels in"=w316, "auto start"=TRUE, "data"=w310, "error in"=w315) -> ("task out"=w319:refnum<k21>, "error out"=w318:errorcluster)  [unwired: 9 in, 1 out]
              n229 = call <vilib>:"DAQmx Wait Until Done.vi"("task/channels in"=w319, "error in"=w318) -> ("task out"=w314:refnum<k21>, "error out"=w313:errorcluster)  [unwired: 12 in]
              n230 = call <vilib>:"DAQmx Clear Task.vi"("task in"=w314, "error in"=w313) -> ("error out"=w311:errorcluster)  [unwired: 13 in]
            }
            event "Swap Memory": Mouse Up {
              n231 = event-data() -> ()  [unwired: 1 in, 1 out]
              n232 = property on="Swap Memory" class="Bool (strict)"("Value"=FALSE ("Swap Memory")) -> ()  [unwired: 2 in, 2 out]
              n233 = flat-sequence {
                tunnel: [w348] -> w335
                tunnel: [w347] -> w334
                tunnel: [w346] -> w333
                tunnel: [w345] -> w332
                tunnel: [w344] -> w331
                tunnel: [w343] -> w330
                tunnel: [w342] -> w329
                tunnel: [w341] -> w328
                tunnel: [w340] -> w326
                tunnel: [w339] -> w325
                tunnel: [w338] -> w324
                tunnel: [w337] -> w323
                tunnel: w335 -> [w354]
                tunnel: w334 -> [w360]
                tunnel: w333 -> [w353]
                tunnel: w332 -> [w359]
                tunnel: w331 -> [w358]
                tunnel: w330 -> [w357]
                tunnel: w329 -> [w356]
                tunnel: w328 -> [w355]
                tunnel: w326 -> [w352]
                tunnel: w325 -> [w351]
                tunnel: w324 -> [w350]
                tunnel: w323 -> [w349]
                frame #0 {
                  n234 = local read "Time of last scan memory"() -> (w346:string)
                  n235 = local read "Info File contents memory"() -> (w348:string)
                  n236 = property on="Memory" class="IntGraph (strict)"() -> ("ZScale.Multiplier"=w344:dbl, "XScale.Ofst&Mult"=w340:T4, "YScale.Ofst&Mult"=w339:T4)  [unwired: 2 in, 2 out]
                  n237 = property on="Image" class="IntGraph (strict)"() -> ("ZScale.Multiplier"=w343:dbl, "XScale.Ofst&Mult"=w338:T4, "YScale.Ofst&Mult"=w337:T4)  [unwired: 2 in, 2 out]
                  n238 = local read "Memory"() -> (w342:dbl[][])
                  n239 = local read "Time of last scan"() -> (w345:string)
                  n240 = local read "Info File contents"() -> (w347:string)
                  n241 = local read "Image"() -> (w341:dbl[][])
                }
                frame #1 {
                  n242 = property on="Image" class="IntGraph (strict)"("ZScale.Multiplier"=w358, "XScale.Ofst&Mult"=w352, "YScale.Ofst&Mult"=w351) -> ()  [unwired: 2 in, 2 out]
                  n243 = property on="Memory" class="IntGraph (strict)"("ZScale.Multiplier"=w357, "XScale.Ofst&Mult"=w350, "YScale.Ofst&Mult"=w349) -> ()  [unwired: 2 in, 2 out]
                  n244 = local write "Image"(w356) -> ()
                  "Info File contents memory" <- w360
                  "Time of last scan memory" <- w359
                  "Memory" <- w355
                  "Info File contents" <- w354
                  "Time of last scan" <- w353
                }
              }
            }
            event "z-Minimum", "z-Maximum", "Step size", "Move to z": Value Change {
              n245 = event-data() -> ()  [unwired: 1 in, 6 out]
              n246 = In Range and Coerce(upper limit=500.0, x="z-Minimum", lower limit=0.0) -> (coerced(x)=w361:dbl)  [unwired: 1 out]
              n247 = local read "Step size"() -> (w367:dbl)
              n248 = In Range and Coerce(upper limit=500.0, x="z-Maximum", lower limit=w361) -> (coerced(x)=w365:dbl)  [unwired: 1 out]
              n249 = Subtract(x=w365, y=w361) -> (x-y=w370:dbl)
              n250 = Divide(x=w370, y=w367) -> (x/y=w369:dbl)
              n251 = Round Toward -Infinity(1:w369) -> (0:w368:dbl)
              n252 = local write "z-Maximum val"(w365) -> ()
              n253 = local write "# steps"(w368) -> ()
              n254 = property on="z-Maximum" class="Slide (strict)"("Value"=w365, "Data Range:Minimum"=w361) -> ()  [unwired: 2 in, 2 out]
              n255 = local write "z-Minimum val"(w361) -> ()
              n256 = local write "z-Minimum"(w361) -> ()
              n257 = local read "Move to z"() -> (w364:bool)
              n258 = case shown="True" w364 {
                tunnel: w363 -> [w375 w377]
                tunnel: [w375 w377] -> w362
                tunnel: w361 -> [_ w376]
                frame False {
                }
                frame True {
                  n259 = local write "requested z-Position"(w376) -> ()
                  n260 = global write "MotorPosition.vi" "Request Z-Position"(w376) -> ()
                }
              }
            }
            event "z-Minimum val", "z-Maximum val": Value Change {
              n261 = event-data() -> ()  [unwired: 1 in, 6 out]
              n262 = local read "z-Minimum val"() -> (w383:dbl)
              n263 = In Range and Coerce(upper limit=500.0, x=w383, lower limit=0.0) -> (coerced(x)=w378:dbl)  [unwired: 1 out]
              n264 = local read "z-Maximum val"() -> (w382:dbl)
              n265 = In Range and Coerce(upper limit=500.0, x=w382, lower limit=w378) -> (coerced(x)=w380:dbl)  [unwired: 1 out]
              n266 = local read "Move to z"() -> (w379:bool)
              n267 = property on="Step size" class="DigNum (strict)"() -> ("Value"=w387:dbl)  [unwired: 2 in, 2 out]
              n268 = Subtract(x=w380, y=w378) -> (x-y=w388:dbl)
              n269 = case shown="True" w379 {
                tunnel: w378 -> [_ w391]
                frame False {
                }
                frame True {
                  n270 = local write "requested z-Position"(w391) -> ()
                  n271 = global write "MotorPosition.vi" "Request Z-Position"(w391) -> ()
                }
              }
              n272 = Divide(x=w388, y=w387) -> (x/y=w386:dbl)
              n273 = Round Toward -Infinity(1:w386) -> (0:w385:dbl)
              n274 = local write "z-Minimum val"(w378) -> ()
              n275 = local write "z-Minimum"(w378) -> ()
              n276 = property on="# Steps" class="DigNum (strict)"("Value"=w385) -> ()  [unwired: 2 in, 2 out]
              n277 = property on="z-Maximum" class="Slide (strict)"("Value"=w380, "Data Range:Minimum"=w378) -> ()  [unwired: 2 in, 2 out]
              n278 = local write "z-Maximum val"(w380) -> ()
            }
            event "Go to white point": Value Change {
              w405 = FALSE ("Go to black point")
              n279 = event-data() -> ()  [unwired: 1 in, 6 out]
              n280 = local read "scaling factor (length/voltage)"() -> (w396:dbl)
              n281 = property on="Image" class="IntGraph (strict)"(error in=w401, "Active Cursor"=u32 2) -> (error out=w402:errorcluster, "Cursor.Cursor Position:Cursor X"=w395:dbl, "Cursor.Cursor Position:Cursor Y"=w393:dbl)  [unwired: 1 in, 1 out]
              n282 = Negate(x=w395) -> (-x=w394:dbl)
              n283 = Negate(x=w393) -> (-x=w392:dbl)
              n284 = Divide(x=w394, y=w396) -> (x/y=w398:dbl)
              n285 = Divide(x=w392, y=w396) -> (x/y=w399:dbl)
              n286 = Build Array(w398, w399) -> (w406:dbl[])
              n287 = call "go_to_point.vi"("error in"=w402, "data"=w406) -> ("error out"=w404:errorcluster)
              n288 = property on="Go to white point" class="Bool (strict)"(error in=w404, "Value"=w405) -> (error out=w403:errorcluster)  [unwired: 1 in, 1 out]
              n289 = property on="Go home" class="Bool (strict)"(error in=w403, "Value"=w405, "Disabled"=T1."Enabled") -> (error out=w400:errorcluster)  [unwired: 1 in, 1 out]
            }
            event "Go home": Value Change {
              n290 = event-data() -> ()  [unwired: 1 in, 6 out]
              n291 = local read "scaling factor (length/voltage)"() -> (w408:dbl)
              n292 = Negate(x="Home X") -> (-x=w411:dbl)
              n293 = Negate(x="Home  Y") -> (-x=w413:dbl)
              n294 = property on="Go home" class="Bool (strict)"("Disabled"=T1."Disabled") -> ()  [unwired: 2 in, 2 out]
              n295 = Divide(x=w411, y=w408) -> (x/y=w409:dbl)
              n296 = Divide(x=w413, y=w408) -> (x/y=w414:dbl)
              n297 = Build Array(w409, w414) -> (w415:dbl[])
              n298 = call "go_to_point.vi"("error in"=w418, "data"=w415) -> ("error out"=w417:errorcluster)
            }
            event "Use white point": Value Change {
              n299 = event-data() -> ()  [unwired: 1 in, 6 out]
              n300 = local read "scaling factor (length/voltage)"() -> (w427:dbl)
              n301 = local read "Field of View"() -> (w432:dbl)
              n302 = Multiply(x=w427, y=w432) -> (x*y=w428:dbl)
              n303 = flat-sequence {
                frame #0 {
                  n304 = Wait (ms)(milliseconds to wait=u32 250) -> ()  [unwired: 1 out]
                }
                frame #1 {
                  n305 = Not(x="Use white point") -> (.not. x?=w440:bool)
                  n306 = property on="Use white point" class="Bool (strict)"("Value"=w440) -> ()  [unwired: 2 in, 2 out]
                }
              }
              n307 = Divide(x=w428, y=2.0) -> (x/y=w419:dbl)
              n308 = property on="Image" class="IntGraph (strict)"("Active Cursor"=u32 2) -> ("Cursor.Cursor Position:Cursor X"=w430:dbl, "Cursor.Cursor Position:Cursor Y"=w429:dbl)  [unwired: 2 in, 2 out]
              n309 = Subtract(x=512.0, y=w419) -> (x-y=w426:dbl)
              n310 = Negate(x=w426) -> (-x=w425:dbl)
              n311 = In Range and Coerce(upper limit=w426, x=w429, lower limit=w425) -> (coerced(x)=w420:dbl)  [unwired: 1 out]
              n312 = In Range and Coerce(upper limit=w426, x=w430, lower limit=w425) -> (coerced(x)=w431:dbl)  [unwired: 1 out]
              n313 = property on="x-Offset" class="DigNum (strict)"("Data Range:Minimum"=w425, "Data Range:Maximum"=w426) -> ()  [unwired: 2 in, 2 out]
              n314 = property on="y-Offset" class="DigNum (strict)"("Data Range:Minimum"=w425, "Data Range:Maximum"=w426) -> ()  [unwired: 2 in, 2 out]
              n315 = local write "x-Offset"(w431) -> ()
              n316 = local write "y-Offset"(w420) -> ()
              n317 = Add(x=w431, y=w419) -> (x+y=w421:dbl)
              n318 = Add(x=w420, y=w419) -> (x+y=w422:dbl)
              n319 = Subtract(x=w431, y=w419) -> (x-y=w423:dbl)
              n320 = Subtract(x=w420, y=w419) -> (x-y=w424:dbl)
              n321 = property on="Image" class="IntGraph (strict)"("Active Cursor"=u32 0, "Cursor.Cursor Position:Cursor X"=w421, "Cursor.Cursor Position:Cursor Y"=w422, "Active Cursor"=u32 1, "Cursor.Cursor Position:Cursor X"=w423, "Cursor.Cursor Position:Cursor Y"=w424) -> ()  [unwired: 2 in, 2 out]
            }
            event "Detector": Value Change {
              n322 = event-data() -> ()  [unwired: 1 in, 6 out]
              n323 = local read "Detector"() -> (w444:u16)
              n324 = case shown="2" w444 {
                tunnel: [T1."Disabled and Grayed Out" ("Disabled") w452 T1."Enabled" ("Disabled")] -> w447
                tunnel: [w449 T1."Enabled" ("Disabled") T1."Enabled" ("Disabled")] -> w445
                tunnel: [w449 w452 T1."Disabled and Grayed Out" ("Disabled")] -> w443
                tunnel: [FALSE TRUE FALSE] -> w442
                frame 0, Default {
                  w449 = T1."Enabled" ("Disabled")
                  # "PMT"
                }
                frame 2 {
                  w452 = T1."Disabled and Grayed Out" ("Disabled")
                  # "OCM"
                }
                frame 1 {
                  # "QEPRo"
                }
              }
              n325 = property on="x-Offset" class="DigNum (strict)"("DisabledEnum"=w445) -> ()  [unwired: 2 in, 2 out]
              n326 = property on="y-Offset" class="DigNum (strict)"("DisabledEnum"=w445) -> ()  [unwired: 2 in, 2 out]
              n327 = property on="Use white point" class="Bool (strict)"("DisabledEnum"=w445) -> ()  [unwired: 2 in, 2 out]
              n328 = property on="Wavelength min" class="DigNum (strict)"("DisabledEnum"=w447) -> ()  [unwired: 2 in, 2 out]
              n329 = property on="Wavelength max" class="DigNum (strict)"("DisabledEnum"=w447) -> ()  [unwired: 2 in, 2 out]
              n330 = property on="Intgration time [us]" class="DigNum (strict)"("DisabledEnum"=w447) -> ()  [unwired: 2 in, 2 out]
              n331 = property on="PMT sensitivity" class="DigNum (strict)"("DisabledEnum"=w443) -> ()  [unwired: 2 in, 2 out]
              n332 = property on="PMT output range" class="Ring (strict)"("DisabledEnum"=w443) -> ()  [unwired: 2 in, 2 out]
              n333 = property on="Scanrate (pixels/s)" class="Ring (strict)"("DisabledEnum"=w443) -> ()  [unwired: 2 in, 2 out]
              n334 = property on="OCM Setup" class="Bool"("Visible"=w442) -> ()  [unwired: 2 in, 2 out]
            }
            event "Quit": Mouse Down {
              n335 = event-data() -> ()  [unwired: 1 in, 8 out]
              n336 = flat-sequence {
                tunnel: w460 -> [w471]
                tunnel: [w462] -> w459
                tunnel: w458 -> [w470]
                tunnel: [w483] -> w461
                tunnel: w459 -> [w483]
                frame #0 {
                  n337 = call-poly <vilib>:"DAQmx Create Virtual Channel.vi"("maximum value"=0.75, "minimum value"=0.0, "physical channels"=tag "Dev1/ao3", "error in"=w471) -> ("task out"=w476:refnum<k21>, "error out"=w475:errorcluster)  [unwired: 10 in]
                  n338 = call-poly <vilib>:"DAQmx Write.vi"("task/channels in"=w476, "auto start"=TRUE, "data"=0.0, "error in"=w475) -> ("task out"=w479:refnum<k21>, "error out"=w478:errorcluster)  [unwired: 9 in, 1 out]
                  n339 = call <vilib>:"DAQmx Wait Until Done.vi"("task/channels in"=w479, "error in"=w478) -> ("task out"=w474:refnum<k21>, "error out"=w473:errorcluster)  [unwired: 12 in]
                  n340 = call <vilib>:"DAQmx Clear Task.vi"("task in"=w474, "error in"=w473) -> ("error out"=w469:errorcluster)  [unwired: 13 in]
                  n341 = invoke class="VI" method="FP.Close"(reference=w470, error in=w469) -> (reference out=w468:refnum<vi>, error out=w467:errorcluster)  [unwired: 1 in, 1 out]
                  n342 = invoke class="VI" method="Ctrl Val.Set"(reference=w468, error in=w467, "Control Name"="QUIT", "Value"=TRUE) -> (reference out=w464:refnum<vi>, error out=w463:errorcluster)  [unwired: 1 in, 3 out]
                  n343 = Close Reference(reference=w464, error in (no error)=w463) -> (error out=w462:errorcluster)
                }
                frame #1 {
                  n344 = Stop() -> ()  [unwired: 1 in]
                }
              }
            }
          }
          n345 = Unbundle By Name(w113) -> ("status"=w110:bool)
          "System" <- w110
          n346 = Not(x=w110) -> (.not. x?=w109:bool)
          n347 = And(x=w109, y="Scan") -> (x .and. y?=w112:bool)
        }
      }
      frame #1 {
        # "These are the info-file contents"
        n348 = local read "Field of View"() -> (w512:dbl)
        n349 = local read "Number of pixels"() -> (w498:i32)
        n350 = Get Date/Time In Seconds() -> (seconds since 1Jan1904=w487:timestamp)
        n351 = local read "x-Offset"() -> (w489:dbl)
        n352 = local read "y-Offset"() -> (w497:dbl)
        n353 = local read "scaling factor (length/voltage)"() -> (w511:dbl)
        n354 = local read "Magnification"() -> (w499:dbl)
        n355 = local read "NA"() -> (w520:dbl)
        n356 = local read "Detector"() -> (w485:u16)
        n357 = local read "PMT sensitivity"() -> (w517:dbl)
        n358 = local read "PMT output range"() -> (w519:dbl)
        n359 = local read "PMT output range"() -> (w521:dbl)
        n360 = local read "Scanrate (pixels/s)"() -> (w518:u32)
        n361 = local read "z-Minimum"() -> (w516:dbl)
        n362 = local read "z-Stacking"() -> (w515:bool)
        n363 = local read "z-Maximum"() -> (w514:dbl)
        n364 = local read "Step size"() -> (w509:dbl)
        n365 = local read "# steps"() -> (w513:u16)
        n366 = local read "xy-Position [µm]"() -> (w506:sgl[])
        n367 = local read "Move to z"() -> (w500:bool)
        n368 = local read "z-Stacking"() -> (w492:bool)
        n369 = local read "Save"() -> (w491:bool)
        n370 = Format Date/Time String(time format string (%c)="%Y-%m-%d, %H%M%S", seconds (now)=w487) -> (date/time string=w486:string)  [unwired: 1 in]
        n371 = Boolean To (0,1)(Boolean=w515) -> (0, 1=w522:i16)
        n372 = Multiply(x=w512, y=w511) -> (x*y=w496:dbl)
        n373 = Not(x=w492) -> (.not. x?=w494:bool)
        n374 = Or(x=w500, y=w492) -> (x .or. y?=w495:bool)
        n375 = And(x=w492, y=w491) -> (x .and. y?=w490:bool)
        n376 = Boolean To (0,1)(Boolean=w494) -> (0, 1=w493:i16)
        n377 = Negate(x=w519) -> (-x=w510:dbl)
        n378 = case shown="True" w490 {
          frame False {
          }
          frame True {
            n379 = local read "File identifier"() -> (w524:string)
            n380 = local read "Time of last scan"() -> (w525:string)
            n381 = Concatenate Strings(w524, w525) -> (w526:string)
            n382 = call "create_directory_structure.vi"("File identifier"=w526) -> ("File path"=w527:path)
            n383 = local write "Path"(w527) -> ()
          }
        }
        n384 = local write "Move to z"(w495) -> ()
        n385 = local write "# steps"(w493) -> ()
        n386 = Index Array(array=w506, index #1=0 ("index"), index #2=1 ("index")) -> (element #1=w503:sgl, element #2=w501:sgl)
        n387 = Boolean To (0,1)(Boolean=w495) -> (0, 1=w502:i16)
        n388 = local read "Intgration time [us]"() -> (w484:u32)
        n389 = Format Into String(format string="%.;%.;Date: %s\nx-offset: %f\ny-offset: %f\nImage Width: %f\nResolution: %d\nobj magn: %d\nNA: %f\nDetector Type: %f\nPMT sensitivity: %f\nDAQ readout min: %f\nDAQ readout max: %f\nScanrate (pixels/s): %d\nz-Minimum: %f\nz-stacking: %u\nz-Maximum: %f\nstep-value: %f\nnumber of steps: %d\nMotor x-pos [µm]: %f\nMotor y-pos [µm]: %f\nMove to z at scan: %u\nIntegration time [us]: %d\n", w486, w489, w497, w496, w498, w499, w520, w485, w517, w510, w521, w518, w516, w522, w514, w509, w513, w503, w501, w502, w484) -> (resulting string=w508:string)  [unwired: 2 in, 1 out]
        n390 = local write "Info File contents"(w508) -> ()
      }
      frame #2 {
        # "The waveforms for the two channels are created"
        n391 = local read "Number of pixels"() -> (w537:i32)
        n392 = Initialize Array(i16 0 ("element"), w537, w537) -> (w539:i16[][])
        n393 = local read "scaling factor (length/voltage)"() -> (w544:dbl)
        n394 = local write "Image"(w539) -> ()
        n395 = call "createScanArrays.vi"("error in"=w550, "resolution"=w537) -> ("error out"=w549:errorcluster, "y-array"=w543:dbl[], "x-array"=w542:dbl[])  [unwired: 3 in]
        n396 = local read "Field of View"() -> (w536:dbl)
        n397 = local read "x-Offset"() -> (w545:dbl)
        n398 = local read "y-Offset"() -> (w532:dbl)
        n399 = Divide(x=w532, y=w544) -> (x/y=w530:dbl)
        n400 = Divide(x=w545, y=w544) -> (x/y=w529:dbl)
        n401 = Multiply(x=w542, y=w536) -> (x*y=w546:dbl[])
        n402 = Multiply(x=w543, y=w536) -> (x*y=w547:dbl[])
        n403 = Multiply(x=w536, y=w544) -> (x*y=w535:dbl)
        n404 = Divide(x=w535, y=2.0) -> (x/y=w531:dbl)
        n405 = Subtract(x=w546, y=w530) -> (x-y=w541:dbl[])
        n406 = Subtract(x=w547, y=w529) -> (x-y=w540:dbl[])
        n407 = Subtract(x=w545, y=w531) -> (x-y=w534:dbl)
        n408 = Subtract(x=w532, y=w531) -> (x-y=w533:dbl)
        n409 = Divide(x=w535, y=w537) -> (x/y=w548:dbl)
        n410 = Build Array(w541, w540) -> (→"scanning waveforms":dbl[][])
        n411 = property on="Image" class="IntGraph (strict)"("X Scale.Offset and Multiplier:Multiplier"=w548, "X Scale.Offset and Multiplier:Offset"=w534, "Y Scale.Offset and Multiplier:Multiplier"=w548, "Y Scale.Offset and Multiplier:Offset"=w533) -> (error out=w553:errorcluster)  [unwired: 2 in, 1 out]
        n412 = property on="Image" class="IntGraph (strict)"(error in=w553) -> ("X Scale.Range:Minimum"=w557:dbl, "Y Scale.Range:Minimum"=w556:dbl, "X Scale.Range:Maximum"=w555:dbl, "Y Scale.Range:Maximum"=w554:dbl)  [unwired: 1 in, 2 out]
        n413 = Subtract(x=w554, y=w556) -> (x-y=w561:dbl)
        n414 = Divide(x=w561, y=2.0) -> (x/y=w559:dbl)
        n415 = Add(x=w559, y=w556) -> (x+y=w558:dbl)
        n416 = Subtract(x=w555, y=w557) -> (x-y=w565:dbl)
        n417 = Divide(x=w565, y=2.0) -> (x/y=w562:dbl)
        n418 = Add(x=w562, y=w557) -> (x+y=w564:dbl)
        n419 = property on="Image" class="IntGraph (strict)"("Active Cursor"=u32 1, "Cursor.Cursor Position:Cursor X"=w557, "Cursor.Cursor Position:Cursor Y"=w556, "Active Cursor"=u32 0, "Cursor.Cursor Position:Cursor X"=w555, "Cursor.Cursor Position:Cursor Y"=w554, "Active Cursor"=u32 2, "Cursor.Cursor Position:Cursor X"=w564, "Cursor.Cursor Position:Cursor Y"=w558) -> ()  [unwired: 2 in, 2 out]
      }
      frame #3 {
        n420 = case shown="1" "Detector" {
          tunnel: [w587 w619] -> w568
          tunnel: w569 -> [w579 w620]
          frame 0, Default {
            w584 = 10348 items=["Volts"=10348, "From Custom Scale"=10065] ("units")
            w592 = 10348 items=["Volts"=10348, "From Custom Scale"=10065] ("units")
            w594 = 10083 items=["default"=-1, "RSE"=10083, "NRSE"=10078, "Differential"=10106, "Pseudodifferential"=12529] ("input terminal configuration")
            w606 = 10178 items=["Finite Samples"=10178, "Continuous Samples"=10123, "Hardware Timed Single Point"=12522] ("sample mode")
            # "Both the writing task (top) and the reading task (bottom) are initialised, but not started yet."
            n421 = local read "scanning waveforms"() -> (w574:dbl[][])
            n422 = Build Array(tag "Dev1/ao1" ("physical channels"), tag "Dev1/ao0" ("physical channels")) -> (w578:tag[])
            n423 = call <vilib>:"DAQmx Flatten Channel String.vi"("names in"=w578, "error in"=w579) -> ("names out"=w575:string, "error out"=w580:errorcluster)  [unwired: 12 in]
            n424 = Array Max & Min(array=w574) -> (max value=w577:dbl, min value=w576:dbl)  [unwired: 2 out]
            n425 = call-poly <vilib>:"DAQmx Create Virtual Channel.vi"("maximum value"=w577, "minimum value"=w576, "physical channels"=w575, "units"=w584, "error in"=w580) -> ("task out"=w581:refnum<k21>, "error out"=w582:errorcluster)  [unwired: 9 in]
            n426 = local read "PMT output range"() -> (w596:dbl)
            n427 = Array Size(array=w574) -> (size(s)=w600:i32[])
            n428 = Negate(x=w596) -> (-x=w595:dbl)
            n429 = local read "Samples/Pixel"() -> (w603:u32)
            n430 = call-poly <vilib>:"DAQmx Create Virtual Channel.vi"("maximum value"=w596, "minimum value"=w595, "input terminal configuration"=w594, "physical channels"=tag "Dev1/ai0", "units"=w592, "error in"=w582) -> ("task out"=w589:refnum<k21>)  [unwired: 8 in, 1 out]
            n431 = Index Array(array=w600, index=1) -> (element=w597:i32)
            n432 = Divide(x=w596, y=32767.0) -> (x/y=w590:dbl)
            n433 = Divide(x=w597, y=2) -> (x/y=w599:dbl)
            n434 = property on="Image" class="IntGraph (strict)"("ZScale.Multiplier"=w590) -> ()  [unwired: 2 in, 2 out]
            n435 = local read "Scanrate (pixels/s)"() -> (w617:u32)
            n436 = Multiply(x=w599, y=w603) -> (x*y=w605:dbl)
            n437 = local read "sampling rate (ADC)"() -> (w571:u32)
            n438 = Max & Min(x=w605, y=u32 25000000) -> (min(x,y)=w608:dbl)  [unwired: 1 out]
            n439 = call <vilib>:"DAQmx Configure Input Buffer.vi"("task/channels in"=w589, "buffer size (in samples per channel)"=w608) -> ("task out"=w615:refnum<k21>, "error out"=w609:errorcluster)  [unwired: 12 in]
            n440 = Multiply(x=w617, y=u32 2) -> (x*y=w602:u32)
            n441 = call-poly <vilib>:"DAQmx Timing.vi"("task/channels in"=w581, "sample mode"=w606, "samples per channel"=w597, "rate"=w602, "error in"=w582) -> ("task out"=w614:refnum<k21>, "error out"=w611:errorcluster)  [unwired: 9 in]
            n442 = call-poly <vilib>:"DAQmx Timing.vi"("task/channels in"=w615, "sample mode"=w606, "samples per channel"=w605, "rate"=w571, "error in"=w609) -> ("task out"=w616:refnum<k21>, "error out"=w607:errorcluster)  [unwired: 9 in]
            n443 = property class="DAQmx Read"(reference=w616, error in=w607, "Read All Available Samples"=TRUE ("ReadAllAvailSamp")) -> (reference out=→"read task":refnum<k21>, error out=w588:errorcluster)
            n444 = call-poly <vilib>:"DAQmx Trigger.vi"("task/channels in"=w614, "source"=tag "/Dev1/ai/StartTrigger", "error in"=w611) -> ("task out"=→"write task":refnum<k21>, "error out"=w572:errorcluster)  [unwired: 11 in]
            n445 = Merge Errors(w572, w588) -> (w587:errorcluster)
          }
          frame 1 {
            w628 = 10348 items=["Volts"=10348, "From Custom Scale"=10065] ("units")
            n446 = local read "scanning waveforms"() -> (w621:dbl[][])
            n447 = Build Array(tag "Dev1/ao1" ("physical channels"), tag "Dev1/ao0" ("physical channels")) -> (w625:tag[])
            n448 = call <vilib>:"DAQmx Flatten Channel String.vi"("names in"=w625, "error in"=w620) -> ("names out"=w622:string, "error out"=w626:errorcluster)  [unwired: 12 in]
            n449 = Array Max & Min(array=w621) -> (max value=w624:dbl, min value=w623:dbl)  [unwired: 2 out]
            n450 = call-poly <vilib>:"DAQmx Create Virtual Channel.vi"("maximum value"=w624, "minimum value"=w623, "physical channels"=w622, "units"=w628, "error in"=w626) -> ("task out"=w618:refnum<k21>, "error out"=w619:errorcluster)  [unwired: 9 in]
            n451 = local write "write task"(w618) -> ()
            n452 = property on="Image" class="IntGraph (strict)"("ZScale.Multiplier"=1.0 ("Z Scale.Offset and Multiplier:Multiplier")) -> ()  [unwired: 2 in, 2 out]
          }
        }
      }
      frame #4 {
        n453 = while {
          tunnel: [w646] -> w633
          shift-right: [w647] -> w632
          shift-left: w631 -> [w650]
          i -> [w642]
          stop <- w648 stop-if-true
          # "This is the recording (looped for z-stacking).\nThe device is read out as fast as possible into a memory buffer,\nwhich is further averaged and transformed to the image."
          n454 = case shown="True" "Move to z" {
            tunnel: w650 -> [w652 w654]
            tunnel: [0.0 ("requested z-Position") w653] -> w634
            tunnel: [w652 w654] -> w636
            frame False {
            }
            frame True {
              # "This moves the stage to the current z-Position"
              n455 = local read "requested z-Position"() -> (w653:dbl)
              n456 = global write "MotorPosition.vi" "Request Z-Position"(w653) -> ()
            }
          }
          n457 = Increment(x=w642) -> (x+1=w640:i32)
          n458 = local read "Info File contents"() -> (w643:string)
          n459 = property on="z-Position" class="DigNum (strict)"("Value"=w634) -> ()  [unwired: 2 in, 2 out]
          n460 = Format Into String(format string="%.;Slide %d z-pos: %f\n", initial string=w643, w640, w634) -> (resulting string=w641:string)  [unwired: 1 in, 1 out]
          n461 = local write "Info File contents"(w641) -> ()
          n462 = flat-sequence {
            tunnel: w636 -> [w657]
            tunnel: [w667] -> w649
            tunnel: [w666] -> w638
            tunnel: [w665] -> w637
            tunnel: [w663] -> w635
            tunnel: w649 -> [w970]
            tunnel: [w971] -> w648
            tunnel: [w965] -> w647
            tunnel: [w969] -> w646
            tunnel: w645 -> [w968]
            tunnel: w638 -> [w966]
            tunnel: w637 -> [w965]
            tunnel: w635 -> [w964]
            frame #0 {
              # "open the shutter"
              n463 = call-poly <vilib>:"DAQmx Create Virtual Channel.vi"("lines"=tag "Dev1/port2/line0", "error in"=w657) -> ("task out"=w661:refnum<k21>, "error out"=w656:errorcluster)  [unwired: 12 in]
              n464 = call-poly <vilib>:"DAQmx Write.vi"("task/channels in"=w661, "data"=TRUE, "error in"=w656) -> ("task out"=w659:refnum<k21>, "error out"=w658:errorcluster)  [unwired: 10 in, 1 out]
              n465 = local read "Detector"() -> (w664:u16)
              n466 = call <vilib>:"DAQmx Clear Task.vi"("task in"=w659, "error in"=w658) -> ("error out"=w655:errorcluster)  [unwired: 13 in]
              n467 = case shown="1" w664 {
                tunnel: [w712 w886] -> w667
                tunnel: [w711 i16[][] []] -> w666
                tunnel: [w689 w845] -> w665
                tunnel: w655 -> [w678 w885]
                tunnel: [u32[][][] [] w868] -> w663
                frame 0, Default {
                  # "Close the shutter"
                  # "Flyback"
                  n468 = local read "Number of pixels"() -> (w709:i32)
                  n469 = local read "scanning waveforms"() -> (w676:dbl[][])
                  n470 = local read "write task"() -> (w679:refnum<k21>)
                  n471 = Initialize Array(0.0 ("element"), w709, w709) -> (w699:dbl[][])
                  n472 = Decrement(x=w709) -> (x-1=w701:i32)
                  n473 = call-poly <vilib>:"DAQmx Write.vi"("task/channels in"=w679, "auto start"=FALSE, "data"=w676, "error in"=w678) -> ("task out"=w682:refnum<k21>, "error out"=w681:errorcluster)  [unwired: 9 in, 1 out]
                  n474 = Divide(x=w709, y=2) -> (x/y=w710:dbl)
                  n475 = Initialize Array(0.0 ("element"), w709, w710) -> (w700:dbl[][])
                  n476 = local read "read task"() -> (w686:refnum<k21>)
                  n477 = call <vilib>:"DAQmx Start Task.vi"("task/channels in"=w682, "error in"=w681) -> ("error out"=w677:errorcluster)  [unwired: 12 in, 1 out]
                  n478 = Obtain Queue(name (unnamed)="Buffer", element data type=i16 0) -> (queue out=w702:refnum<queue>)  [unwired: 3 in, 2 out]
                  n479 = Negate(x=w710) -> (-x=w703:dbl)
                  n480 = call <vilib>:"DAQmx Start Task.vi"("task/channels in"=w686, "error in"=w677) -> ("task out"=w684:refnum<k21>, "error out"=w685:errorcluster)  [unwired: 12 in]
                  n481 = while {
                    shift-right: [w759] -> _
                    shift-left: w701 -> [w763]
                    shift-right: [w752] -> _
                    shift-left: w701 -> [w762]
                    tunnel: w701 -> [w761]
                    shift-right: [w760] -> w712
                    shift-left: w699 -> [w764]
                    shift-right: [w758] -> w691
                    shift-left: w685 -> [w748]
                    tunnel: w703 -> [w757]
                    tunnel: w702 -> [w746]
                    shift-right: [w741] -> w711
                    shift-left: w700 -> [w742]
                    stop <- w754 stop-if-true
                    # "x-counter"
                    # "y-counter"
                    n482 = local read "Samples/Pixel"() -> (w750:u32)
                    n483 = Get Queue Status(queue=w746, error in (no error)=w748) -> (queue out=w745:refnum<queue>, error out=w749:errorcluster, # elements in queue=w747:i32)  [unwired: 1 in, 5 out]
                    n484 = Greater Or Equal?(x=w747, y=w750) -> (x >= y?=w765:bool)
                    n485 = case shown="True" w765 {
                      tunnel: w749 -> [w768 w779]
                      tunnel: w750 -> [_ w776]
                      tunnel: w764 -> [w769 w790]
                      tunnel: w763 -> [w771 w780]
                      tunnel: w762 -> [w770 w788]
                      tunnel: w761 -> [_ w787]
                      tunnel: [w769 w786] -> w760
                      tunnel: [w771 w785] -> w759
                      tunnel: [w770 w784] -> w752
                      tunnel: [w768 w778] -> w758
                      tunnel: w757 -> [_ w782]
                      tunnel: w745 -> [_ w777]
                      tunnel: [bool[] [FALSE] w774] -> w744
                      tunnel: w742 -> [w766 w773]
                      tunnel: [w766 w772] -> w741
                      frame False {
                      }
                      frame True {
                        n486 = for {
                          N: w776 -> [_]
                          tunnel: w777 -> [w793]
                          shift-right: [w794] -> w778
                          shift-left: w779 -> [w795]
                          tunnel: [w792] -> w775 mode=indexing
                          tunnel: [w791] -> w774 mode=indexing
                          n487 = Dequeue Element(queue=w793, error in (no error)=w795) -> (element=w792:i16, timed out?=w791:bool, error out=w794:errorcluster)  [unwired: 1 in, 1 out]
                        }
                        n488 = Greater Or Equal To 0?(x=w780) -> (x >= 0?=w781:bool)
                        n489 = Equal?(x=w782, y=w780) -> (x = y?=w783:bool)
                        n490 = Decrement(x=w780) -> (x-1=w789:i32)
                        n491 = case shown="False" w781 {
                          tunnel: w775 -> [w801 w810]
                          tunnel: w790 -> [w805 w816]
                          tunnel: w788 -> [w800 w813]
                          tunnel: [w805 w815] -> w786
                          tunnel: w780 -> [w798 w814]
                          tunnel: w773 -> [w802 w807]
                          tunnel: [w803 w807] -> w772
                          frame False {
                            n492 = Negate(x=w798) -> (-x=w799:i32)
                            n493 = call-poly <vilib>:"Mean.vi"("X"=w801) -> ("mean"=w804:dbl)  [unwired: 1 out]
                            n494 = Decrement(x=w799) -> (x-1=w797:i32)
                            n495 = Negate(x=w804) -> (-x=w796:dbl)
                            n496 = Replace Array Subset(array=w802, new element=w796, index (row)=w800, index (col)=w797) -> (w803:dbl[][])
                          }
                          frame True {
                            n497 = local read "Throw away"() -> (w809:bool)
                            n498 = case shown="True" w809 {
                              tunnel: w810 -> [w817 w820]
                              tunnel: [w817 w819] -> w811
                              frame False {
                              }
                              frame True {
                                n499 = local read "Thrown samples"() -> (w818:i16)
                                n500 = Array Subset(array=w820, index=w818) -> (w819:i16[])  [unwired: 1 in]
                              }
                            }
                            n501 = call-poly <vilib>:"Mean.vi"("X"=w811) -> ("mean"=w808:dbl)  [unwired: 1 out]
                            n502 = Negate(x=w808) -> (-x=w806:dbl)
                            n503 = To Word Integer(number=w806) -> (16bit integer=w812:i16)
                            n504 = Replace Array Subset(array=w816, new element=w812, index (row)=w813, index (col)=w814) -> (w815:dbl[][])
                          }
                        }
                        n505 = case shown="True" w783 {
                          tunnel: w788 -> [w822 w835]
                          tunnel: [w822 w834] -> w784
                          tunnel: w786 -> [_ w825]
                          tunnel: [w821 w836] -> w785
                          tunnel: w789 -> [w821 _]
                          tunnel: w787 -> [_ w836]
                          frame False {
                          }
                          frame True {
                            n506 = local read "Time per line [s]"() -> (w824:dbl)
                            n507 = Multiply(x=w824, y=w835) -> (x*y=w827:dbl)
                            n508 = Decrement(x=w835) -> (x-1=w834:i32)
                            n509 = Quotient & Remainder(x=w827, y=60.0) -> (x-y*floor(x/y)=w830:dbl, floor(x/y)=w832:dbl)
                            n510 = Divide(x=w830, y=100.0) -> (x/y=w831:dbl)
                            n511 = Add(x=w831, y=w832) -> (x+y=w828:dbl)
                            n512 = Number To Fractional String(number=w828, precision (6)=i16 2) -> (F-format string=w823:string)  [unwired: 2 in]
                            n513 = local write "Duration (m.s)"(w823) -> ()
                            "Image" <- w825
                          }
                        }
                      }
                    }
                    n514 = Or Array Elements(Boolean array=w744) -> (logical OR=w743:bool)
                    n515 = local read "Scan"() -> (w751:bool)
                    n516 = Not(x=w751) -> (.not. x?=w753:bool)
                    n517 = Unbundle By Name(w758) -> ("status"=w756:bool)
                    n518 = Less Than 0?(x=w752) -> (x < 0?=w755:bool)
                    n519 = Compound Arithmetic op=OR(w756, w755, w753, w743) -> (w754:bool)
                  }
                  n520 = while {
                    shift-right: [w722] -> w690
                    shift-left: w685 -> [w735]
                    tunnel: w702 -> [w721]
                    tunnel: [w714] -> w687
                    tunnel: w684 -> [w713]
                    stop <- w733 stop-if-true
                    w734 = -1.0 ("timeout")
                    n521 = call-poly <vilib>:"DAQmx Read.vi"("task/channels in"=w713, "number of samples per channel"=w734, "timeout"=w734, "error in"=w735) -> ("task out"=w730:refnum<k21>, "data"=w717:i16[], "error out"=w720:errorcluster)  [unwired: 9 in]
                    n522 = Array Size(array=w717) -> (size(s)=w718:i32)
                    n523 = for {
                      N: w718 -> [_]
                      tunnel: w721 -> [w740]
                      shift-right: [w738] -> w719
                      shift-left: w720 -> [w739]
                      tunnel: w717 -> [w737] mode=indexing
                      tunnel: [w736] -> w716 mode=indexing
                      n524 = Enqueue Element(queue=w740, element=w737, error in (no error)=w739) -> (timed out?=w736:bool, error out=w738:errorcluster)  [unwired: 1 in, 1 out]
                    }
                    n525 = Or Array Elements(Boolean array=w716) -> (logical OR=w715:bool)
                    n526 = call <vilib>:"DAQmx Is Task Done.vi"("task/channels in"=w730, "error in"=w719) -> ("task out"=w725:refnum<k21>, "task done?"=w727:bool, "error out"=w724:errorcluster)  [unwired: 11 in]
                    n527 = property class="DAQmx Read"(reference=w725, error in=w724) -> (reference out=w714:refnum<k21>, error out=w722:errorcluster, "AvailSampPerChan"=w729:u32)
                    n528 = Equal To 0?(x=w729) -> (x = 0?=w728:bool)
                    n529 = local read "Scan"() -> (w723:bool)
                    n530 = And(x=w728, y=w727) -> (x .and. y?=w726:bool)
                    n531 = Unbundle By Name(w722) -> ("status"=w732:bool)
                    n532 = Not(x=w723) -> (.not. x?=w731:bool)
                    n533 = Compound Arithmetic op=OR(w732, w731, w726, w715) -> (w733:bool)
                  }
                  n534 = call <vilib>:"DAQmx Stop Task.vi"("task/channels in"=w687, "error in"=w690) -> ("error out"=w669:errorcluster)  [unwired: 12 in, 1 out]
                  n535 = local read "write task"() -> (w698:refnum<k21>)
                  n536 = call <vilib>:"DAQmx Stop Task.vi"("task/channels in"=w698, "error in"=w691) -> ("error out"=w688:errorcluster)  [unwired: 12 in, 1 out]
                  n537 = call-poly <vilib>:"DAQmx Create Virtual Channel.vi"("lines"=tag "Dev1/port2/line0", "error in"=w669) -> ("task out"=w671:refnum<k21>, "error out"=w672:errorcluster)  [unwired: 12 in]
                  n538 = call-poly <vilib>:"DAQmx Write.vi"("task/channels in"=w671, "data"=FALSE, "error in"=w672) -> ("task out"=w674:refnum<k21>, "error out"=w675:errorcluster)  [unwired: 10 in, 1 out]
                  n539 = call <vilib>:"DAQmx Clear Task.vi"("task in"=w674, "error in"=w675) -> ("error out"=w668:errorcluster)  [unwired: 13 in]
                  n540 = Merge Errors(w688, w669, w668) -> (w692:errorcluster)
                  n541 = Obtain Queue(name (unnamed)="Buffer", element data type=i16 0, error in (no error)=w692) -> (queue out=w695:refnum<queue>, error out=w693:errorcluster)  [unwired: 2 in, 1 out]
                  n542 = Release Queue(queue=w695, force destroy? (F)=TRUE, error in (no error)=w693) -> (error out=w689:errorcluster)  [unwired: 2 out]
                }
                frame 1 {
                  # "Close the shutter"
                  # "Flyback"
                  n543 = local read "Number of pixels"() -> (w871:i32)
                  n544 = local read "scanning waveforms"() -> (w841:dbl[][])
                  n545 = call "Maya2000 - Open all.vi"() -> ("error out"=w882:errorcluster, ".NET Refnum out"=w884:refnum<k24>, "Maya2000 Basic \n[UV2400,UV600]"=w883:T5[])  [unwired: 9 in]
                  n546 = call "Maya2000 - set N coadd and integr time.vi"("Intgration time\n[us]"="Intgration time [us]", "error in (no error)"=w882, "Maya2000 basic values"=w883, ".NET Refnum in"=w884) -> ("error out"=w878:errorcluster, "This instruments index"=w875:i32, ".NET Refnum out"=w877:refnum<k24>)  [unwired: 4 in, 1 out]
                  n547 = Initialize Array(0.0 ("element"), w871, w871) -> (w887:dbl[][])
                  n548 = Decrement(x=w871) -> (x-1=w873:i32)
                  n549 = invoke class="NETWrapper" method="getWavelengths"(reference=w877, error in=w878, "spectrometerIndex"=w875) -> (reference out=w876:refnum<k24>, error out=w874:errorcluster, "getWavelengths"=w858:dbl[])  [unwired: 1 in, 1 out]
                  n550 = Array Size(array=w858) -> (size(s)=w869:i32)
                  n551 = Initialize Array(u32 0 ("element"), w871, w871, w869) -> (w870:u32[][][])
                  n552 = Divide(x=w871, y=2) -> (x/y=w891:dbl)
                  n553 = Negate(x=w891) -> (-x=w888:dbl)
                  n554 = Subtract(x=w858, y="Wavelength min") -> (x-y=w863:dbl[])
                  n555 = Subtract(x=w858, y="Wavelength max") -> (x-y=w860:dbl[])
                  n556 = Index Array(array=w841, index (row)=0) -> (element=w838:dbl[])  [unwired: 1 in]
                  n557 = Index Array(array=w841, index (row)=1) -> (element=w837:dbl[])  [unwired: 1 in]
                  n558 = Absolute Value(x=w863) -> (abs(x)=w862:dbl[])
                  n559 = Absolute Value(x=w860) -> (abs(x)=w859:dbl[])
                  n560 = Array Max & Min(array=w862) -> (min index (indices)=w857:i32)  [unwired: 3 out]
                  n561 = Array Max & Min(array=w859) -> (min index (indices)=w856:i32)  [unwired: 3 out]
                  n562 = Decimate 1D Array(w838) -> (w866:dbl[])  [unwired: 1 out]
                  n563 = Decimate 1D Array(w837) -> (w865:dbl[])  [unwired: 1 out]
                  n564 = Subtract(x=w856, y=w857) -> (x-y=w855:i32)
                  n565 = for {
                    tunnel: w888 -> [w927]
                    shift-right: [w910] -> w843
                    shift-left: w885 -> [w902]
                    tunnel: w876 -> [w909]
                    tunnel: w875 -> [w908]
                    tunnel: [w907] -> w879
                    tunnel: w874 -> [_]
                    shift-right: [w917] -> w886
                    shift-left: w887 -> [w924]
                    shift-right: [w921] -> _
                    shift-left: w873 -> [w925]
                    tunnel: w873 -> [w918]
                    shift-right: [w919] -> _
                    shift-left: w873 -> [w920]
                    shift-right: [w911] -> w868
                    shift-left: w870 -> [w912]
                    tunnel: w866 -> [w904] mode=indexing
                    tunnel: w865 -> [w903] mode=indexing
                    tunnel: w857 -> [w906]
                    tunnel: w855 -> [w905]
                    stop <- w914 stop-if-true
                    # "x-counter"
                    # "y-counter"
                    n566 = Equal?(x=w927, y=w925) -> (x = y?=w923:bool)
                    n567 = Decrement(x=w925) -> (x-1=w922:i32)
                    n568 = Greater Or Equal To 0?(x=w925) -> (x >= 0?=w926:bool)
                    n569 = local read "write task"() -> (w900:refnum<k21>)
                    n570 = Build Array(w904, w903) -> (w899:dbl[])
                    n571 = call-poly <vilib>:"DAQmx Write.vi"("task/channels in"=w900, "auto start"=TRUE, "data"=w899, "error in"=w902) -> ("number of samples written per channel"=w897:u32, "error out"=w901:errorcluster)  [unwired: 9 in, 1 out]
                    n572 = local read "Intgration time [us]"() -> (w893:u32)
                    n573 = Divide(x=w893, y=u32 1000) -> (x/y=w894:dbl)
                    n574 = Multiply(x=w894, y=w897) -> (x*y=w895:dbl)
                    n575 = Wait (ms)(milliseconds to wait=w895) -> (millisecond timer value=w896:u32)
                    n576 = case shown="True" w926 {
                      tunnel: w925 -> [_ w959]
                      tunnel: w920 -> [_ w960]
                      tunnel: w924 -> [w947 w963]
                      tunnel: [w947 w962] -> w917
                      tunnel: w912 -> [w946 w961]
                      tunnel: [w946 w958] -> w911
                      tunnel: w901 -> [w944 w956]
                      tunnel: [w944 w955] -> w910
                      tunnel: w909 -> [w945 w954]
                      tunnel: w908 -> [_ w953]
                      tunnel: [w945 w952] -> w907
                      tunnel: w906 -> [_ w949]
                      tunnel: w905 -> [_ w948]
                      tunnel: w896 -> [_ _]
                      frame False {
                      }
                      frame True {
                        n577 = invoke class="NETWrapper" method="getSpectrum"(reference=w954, error in=w956, "spectrometerIndex"=w953) -> (reference out=w952:refnum<k24>, error out=w955:errorcluster, "getSpectrum"=w951:dbl[])  [unwired: 1 in, 1 out]
                        n578 = Replace Array Subset(array=w961, new element=w951, index (dim 0)=w960, index (dim 1)=w959) -> (w958:u32[][][])  [unwired: 1 in]
                        n579 = Array Subset(array=w951, index=w949, length=w948) -> (w950:dbl[])
                        n580 = call-poly <vilib>:"Mean.vi"("X"=w950) -> ("mean"=w957:dbl)  [unwired: 1 out]
                        n581 = Replace Array Subset(array=w963, new element=w957, index (row)=w960, index (col)=w959) -> (w962:dbl[][])
                      }
                    }
                    n582 = case shown="True" w923 {
                      tunnel: w922 -> [w929 _]
                      tunnel: [w929 w942] -> w921
                      tunnel: w920 -> [w928 w933]
                      tunnel: [w928 w943] -> w919
                      tunnel: w918 -> [_ w942]
                      tunnel: w917 -> [_ w930]
                      frame False {
                      }
                      frame True {
                        n583 = local read "Time per line [s]"() -> (w931:dbl)
                        n584 = Decrement(x=w933) -> (x-1=w943:i32)
                        n585 = Multiply(x=w931, y=w933) -> (x*y=w935:dbl)
                        n586 = Quotient & Remainder(x=w935, y=60.0) -> (x-y*floor(x/y)=w938:dbl, floor(x/y)=w940:dbl)
                        n587 = Divide(x=w938, y=100.0) -> (x/y=w939:dbl)
                        n588 = Add(x=w939, y=w940) -> (x+y=w936:dbl)
                        n589 = Number To Fractional String(number=w936, precision (6)=i16 2) -> (F-format string=w932:string)  [unwired: 2 in]
                        n590 = local write "Duration (m.s)"(w932) -> ()
                        n591 = local write "Image"(w930) -> ()
                      }
                    }
                    n592 = local read "Scan"() -> (w916:bool)
                    n593 = Unbundle By Name(w910) -> ("status"=w913:bool)
                    n594 = Not(x=w916) -> (.not. x?=w915:bool)
                    n595 = Or(x=w913, y=w915) -> (x .or. y?=w914:bool)
                  }
                  n596 = local read "write task"() -> (w844:refnum<k21>)
                  n597 = call "Maya2000 - Close all.vi"("error in (no error)"=w843, "Maya reference in"=w879) -> ("error out"=w881:errorcluster, ".NET Refnum out"=w880:refnum<k24>)  [unwired: 8 in]
                  n598 = call <vilib>:"DAQmx Stop Task.vi"("task/channels in"=w844, "error in"=w843) -> ("error out"=w842:errorcluster)  [unwired: 12 in, 1 out]
                  n599 = call-poly <vilib>:"DAQmx Create Virtual Channel.vi"("lines"=tag "Dev1/port2/line0", "error in"=w843) -> ("task out"=w849:refnum<k21>, "error out"=w850:errorcluster)  [unwired: 12 in]
                  n600 = Close Reference(reference=w880, error in (no error)=w881) -> (error out=w846:errorcluster)
                  n601 = call-poly <vilib>:"DAQmx Write.vi"("task/channels in"=w849, "data"=FALSE, "error in"=w850) -> ("task out"=w852:refnum<k21>, "error out"=w853:errorcluster)  [unwired: 10 in, 1 out]
                  n602 = call <vilib>:"DAQmx Clear Task.vi"("task in"=w852, "error in"=w853) -> ("error out"=w847:errorcluster)  [unwired: 13 in]
                  n603 = Merge Errors(w846, w847, w842) -> (w845:errorcluster)
                }
              }
            }
            frame #1 {
              n604 = local read "requested z-Position"() -> (w979:dbl)
              n605 = local read "Step size"() -> (w978:dbl)
              n606 = local read "z-Maximum"() -> (w977:dbl)
              n607 = local read "Save"() -> (w976:bool)
              n608 = Add(x=w978, y=w979) -> (x+y=w972:dbl)
              n609 = Greater?(x=w972, y=w977) -> (0:w974:bool)
              n610 = local read "z-Stacking"() -> (w980:bool)
              n611 = And(x=w968, y=w976) -> (x .and. y?=w975:bool)
              n612 = Not(x=w974) -> (.not. x?=w981:bool)
              n613 = And(x=w980, y=w981) -> (x .and. y?=w973:bool)
              n614 = Not(x=w980) -> (.not. x?=w982:bool)
              n615 = case shown="True" w973 {
                tunnel: w972 -> [_ w987]
                tunnel: [w985 w986] -> w967
                frame False {
                  n616 = local read "# steps"() -> (w985:u16)
                }
                frame True {
                  n617 = local write "requested z-Position"(w987) -> ()
                  n618 = local read "# steps"() -> (w986:u16)
                  n619 = Increment(x=w986) -> (x+1=w988:u16)
                  n620 = local write "# steps"(w988) -> ()
                }
              }
              n621 = local read "Scan"() -> (w969:bool)
              n622 = Unbundle By Name(w965) -> ("status"=w984:bool)
              n623 = Not(x=w969) -> (.not. x?=w983:bool)
              n624 = Compound Arithmetic op=OR(w984, w983, w982, w974) -> (w971:bool)
              n625 = case shown="True" w975 {
                tunnel: w970 -> [_ w996]
                tunnel: w971 -> [_ w994]
                tunnel: w967 -> [_ w989]
                tunnel: w966 -> [_ w993]
                tunnel: w964 -> [_ w991]
                frame False {
                }
                frame True {
                  n626 = local read "Detector"() -> (w990:u16)
                  n627 = local read "Info File contents"() -> (w997:string)
                  n628 = local read "Additional info"() -> (w999:string)
                  n629 = Concatenate Strings("info: " ("string"), w999, "\n", w997) -> (w995:string)
                  n630 = local read "Path"() -> (w992:path)
                  n631 = case shown="1" w990 {
                    tunnel: w992 -> [_ w1008]
                    tunnel: w991 -> [_ w1006]
                    tunnel: w989 -> [_ w1003]
                    frame 0, Default {
                    }
                    frame 1 {
                      n632 = Path To String(path=w1008) -> (string=w1002:string)
                      n633 = Number To Decimal String(number=w1003) -> (decimal integer string=w1004:string)  [unwired: 1 in]
                      n634 = Concatenate Strings(w1002, "_" ("string"), w1004, "_spectrum.dat" ("string")) -> (w1011:string)
                      n635 = String To Path(string=w1011) -> (path=w1007:path)
                      n636 = Write to Binary File(file (use dialog)=w1007, data=w1006) -> (refnum out=w1009:refnum<file>, error out=w1010:errorcluster)  [unwired: 4 in, 1 out]
                      n637 = Close File(refnum=w1009, error in=w1010) -> ()  [unwired: 2 out]
                    }
                  }
                  n638 = call "save_to_disk.vi"("Retrace"=w993, "slice"=w989, "write info file?"=w994, "Scan info"=w995, "Image"=w996, "File path"=w992) -> ()  [unwired: 3 in, 1 out]
                }
              }
              "Retrace" <- w966
              "spectral image" <- w964
            }
          }
          n639 = local read "z-Stacking"() -> (w645:bool)
        }
      }
      frame #5 {
        w1024 = path "M:/Data/scan.log" ("path to log")
        # "The device is cleared, the cursors are moved to the image edge.\nThe log-file is updated."
        n640 = case shown="False" w1019 {
          tunnel: w1024 -> [w1035 w1040]
          frame False {
            n641 = Get Date/Time In Seconds() -> (seconds since 1Jan1904=w1033:timestamp)
            n642 = Format Into String(format string="%T: Scan stopped\\n", w1033) -> (resulting string=w1032:string)  [unwired: 2 in, 1 out]
            n643 = call <vilib>:"Write Characters To File.vi"("append to file? (new file:F)"=TRUE, "character string"=w1032, "file path (dialog if empty)"=w1035) -> ()  [unwired: 2 in, 1 out]
          }
          frame True {
            n644 = Get Date/Time In Seconds() -> (seconds since 1Jan1904=w1038:timestamp)
            n645 = Format Into String(format string="%<%Y-%m-%d %H:%M:%S>T: Slice scan finished\\n", w1038) -> (resulting string=w1037:string)  [unwired: 2 in, 1 out]
            n646 = call <vilib>:"Write Characters To File.vi"("append to file? (new file:F)"=TRUE, "character string"=w1037, "file path (dialog if empty)"=w1040) -> ()  [unwired: 2 in, 1 out]
          }
        }
        n647 = Unbundle By Name(w1016) -> ("status"=w1021:bool, "code"=w1022:i32, "source"=w1023:string)
        n648 = case shown="False" w1021 {
          tunnel: w1022 -> [_ w1026]
          tunnel: w1023 -> [_ w1025]
          tunnel: w1024 -> [_ w1030]
          frame False {
          }
          frame True {
            n649 = Get Date/Time In Seconds() -> (seconds since 1Jan1904=w1027:timestamp)
            n650 = Format Into String(format string="%<%Y-%m-%d %H:%M:%S>T: Error encountered: %d: %s. Scan will abort.\\n", w1027, w1026, w1025) -> (resulting string=w1028:string)  [unwired: 2 in, 1 out]
            n651 = call <vilib>:"Write Characters To File.vi"("append to file? (new file:F)"=TRUE, "character string"=w1028, "file path (dialog if empty)"=w1030) -> ()  [unwired: 2 in, 1 out]
          }
        }
        n652 = local read "write task"() -> (w1013:refnum<k21>)
        n653 = local read "read task"() -> (w1012:refnum<k21>)
        n654 = call <vilib>:"DAQmx Clear Task.vi"("task in"=w1013) -> ("error out"=w1015:errorcluster)  [unwired: 14 in]
        n655 = call <vilib>:"DAQmx Clear Task.vi"("task in"=w1012) -> ("error out"=w1014:errorcluster)  [unwired: 14 in]
        n656 = Merge Errors(w1016, w1015, w1014) -> (w1017:errorcluster)
        n657 = Unbundle By Name(w1017) -> ("status"=w1020:bool)
        n658 = local write "System"(w1020) -> ()
        n659 = local write "Scan"(FALSE ("Scan")) -> ()
      }
    }
  }
  n660 = call <vilib>:"Simple Error Handler.vi"("error in (no error)"=w19) -> ()  [unwired: 4 in, 5 out]
